vi "COD主界面（列队使用）.vi"() -> (8 "多列列表框":i32(listbox))   [LabVIEW 2016, in "斯坦道CODMn.lvlib"]
uses:
  <vilib>/Analysis/6fits.llb/Curve Fitting Criteria.ctl
  <vilib>/Utility/miscctls.llb/LVPointTypeDef.ctl
  <vilib>/Plasmionique/MB Master/MB_Master_Serial/MB_Master_Serial.lvclass
  D:/Program Files (x86)/National Instruments/LabVIEW 2016/vi.lib/Plasmionique/MB Master/MB_Master/MB_Master.lvclass
  <vilib>/Utility/config.llb/Read Key (Double).vi
  <vilib>/Utility/config.llb/Read Key (U32).vi
  <vilib>/Utility/config.llb/Write Key (Double).vi
  <vilib>/Utility/config.llb/Read Key (I32).vi
  <vilib>/Utility/config.llb/Read Key (Boolean).vi
  <vilib>/Utility/config.llb/Write Key (Boolean).vi
  <vilib>/Utility/config.llb/Write Key (I32).vi
  <vilib>/Waveform/WDTFileIO.llb/Read Waveform from File.vi
  <vilib>/Plasmionique/MB Master/MB Master.lvlib
  <vilib>/ptbypt/NI_PtbyPt.lvlib
  <vilib>/Utility/config.llb/NI_LVConfig.lvlib
  <vilib>/Analysis/NI_AALPro.lvlib
panel:
  out "基本量程(显示)":string
  out "测量模式(显示)":string
  in  "量程切换次数":u8
  in  "CODMn空白测试选择":enum16{"空白测试走纯水管", "空白测试走标样管"}(ring)
  out "数据时间":string
  out "断电排液标记":bool
  in  "测量模式":T1(ring)
  in  "高切低阈值":dbl
  in  "低切高阈值":dbl
  out "COM":string
  in  "启用5":bool
  in  "校准5":bool
  in  "泵滴定数5":dbl
  in  "浓度5":dbl
  in  "启用4":bool
  in  "校准4":bool
  in  "泵滴定数4":dbl
  in  "浓度4":dbl
  out "波形时间":timestamp
  in  "历史波形":bool
  out "滴定数-ORP值":u16[](array[numeric]) caption="数组"
  in  "关闭 3":bool
  in  "滴定曲线":bool
  out "ORP滴定曲线2":u16[](graph)
  in  "跨度液浓度":dbl
  out "空白测试标记":bool
  out "跨度核查标记":bool
  out "启动选择 2":u16(ring) items=["水样测试", "标样核查", "零点核查", "跨度核查", "空白测试", "加标回收", "平行样", "校零", "校标"]
  in  "量程选择":enum16{"低量程", "高量程", "0-2量程"}(ring)
  in  "手动控制":bool
  in  "选用水样":enum16{"葡萄糖", "草酸钠"}(ring)
  in  "方程系数":cluster{"X^2":dbl, "X":dbl, "b":dbl} {"X^2" format="%#.6g"; "b" format="%#.6g"; "X" format="%#.6g"}
  out "多项式系数1":dbl[](array[numeric]) caption="多项式系数"
  out "XY图":cluster{"X Values":dbl[], "Y Values":dbl[]}[](graph)
  in  "模型":enum32{"线性", "多项式"}(ring)
  out "启动时间":timestamp format="%<%Y/%m/%d %H:%M:%S>T"
  in  "自动切换量程":enum16{"关闭", "自动切换测一次", "自动切换测两次"}(ring)
  in  "24H周期设置":bool[](xcontrol)
  in  "关闭 2":bool
  in  "周期设置":bool
  out "文本.文本":string
  out "r^2":dbl format="%.8g"
  out "拟合公式":string
  out "b":dbl format="%#.4g"
  out "K":dbl format="%#.4f"
  out "当前校准":i32
  in  "启用3":bool
  in  "启用2":bool
  in  "启用1":bool
  in  "校准3":bool
  in  "校准2":bool
  in  "校准1":bool
  in  "泵滴定数3":dbl
  in  "泵滴定数2":dbl
  in  "泵滴定数1":dbl
  in  "浓度3":dbl
  in  "浓度2":dbl
  in  "浓度1":dbl
  in  "写入":bool
  out "测量模式数字":i32
  out "零点核查标记":bool
  out "排液故障":bool
  out "进水样超量程":bool
  out "标样核查标记":bool
  out "平行样测量":bool
  out "加标回收测量":bool
  out "质控样测量":bool
  out "待机":bool
  out "校标错误":bool
  out "校零错误":bool
  out "测量错误":bool
  out "草酸钠报警":bool
  out "高锰酸钾报警":bool
  out "加热故障":bool
  out "温控器故障":bool
  out "ORP故障":bool
  out "排液标记":bool
  out "故障标记":bool
  out "校标标记":bool
  out "校零标记":bool
  out "通讯状态":bool
  out "水样测量":bool
  out "读取KB值":bool
  in  "读取":bool
  in  "返回":bool
  in  "校准配置":bool
  in  "修正系数 2":dbl
  in  "浓度 2":dbl
  in  "温度":dbl
  in  "恒温时间":dbl
  in  "基本量程":enum16{"10mg/L", "20mg/L"}(ring)
  in  "水样":dbl
  in  "蒸馏水":dbl
  in  "标液":dbl
  in  "质控样":dbl
  in  "加标回收":dbl
  in  "草酸钠":dbl
  in  "高锰酸钾":dbl
  in  "硫酸":dbl
  in  "零点泵计量数 2":dbl
  in  "标度泵计量数 2":dbl
  out "标度滴定值":dbl
  out "零点滴定值":dbl
  in  "保存":bool
  in  "关闭":bool
  out "测量数据区":T2 {"单位" items=["ug/L", "mg/L", "ppm", "mg/m3", "cm", "ppb", "ug/m3", "%", "nmol/mol", "umol/mol", "MPN/L", "MPN/100ml", "ng/m3", "NTU", "无量纲", "ms/cm", "us/cm", "℃", "mV", "万个/L"]}
  out "仪器时间":timestamp format="%<%Y/%m/%d %H:%M:%S>T"
  out "秒":u16
  out "分":u16
  out "COD浓度（mg/L)":dbl format="%.2g"
  out "进样管":dbl
  out "高锰酸钾":dbl
  out "草酸钠":dbl
  out "硫酸":dbl
  out "ORP显示":dbl
  out "温度":dbl
  out "加热":bool
  out "搅拌":bool
  out "进硫酸":bool
  out "进加标回收样":bool
  out "进质控样":bool
  out "进标液":bool
  out "进蒸馏水":bool
  out "进水样":bool
  out "进草酸钠":bool
  out "进高锰酸钾":bool
  out "定时启动":bool
  in  "启动":bool
  in  "故障清除":bool
  in  "参数配置":bool
  in  "停止":bool
  in  "单步启动":bool
  out "系统时间":timestamp
  in  "时间校准":bool
  in  "枚举":enum16{"读取数据", "写入数据", "读取写入DATABASE", "读取参数"}(ring)
  out "报警簇":T3
  out "Registers":u16[](array[numeric])
  in  "Slave ID":u8=1
  in  "Serial Config":T4={"baud rate (bps)"=115200, "stop bits"=10, "parity"=0, "flow control"=0, "timeout"=1000, "retries"=1} {"stop bits" items=["1.0"=10, "1.5"=15, "2.0"=20]; "flow control" items=["None", "XON/XOFF", "RTS/CTS", "XON/XOFF & RTS/CTS", "DTR/DSR", "XON/XOFF & DTR/DSR"]; "parity" items=["None", "Odd", "Even", "Mark", "Space"]}
  in  "温度 2":dbl
  in  "浓度":dbl
  in  "修正系数":dbl
  in  "标样浓度 2":dbl
  out "模式（受控）":u16
  in  "VISA resource name":refnum<visa-resource-name>="COM4" caption="VISA资源名称"
  # "测量时间："
  # "水样~加标回收"
  # "mV"
  # "℃"
  # "注：遇到加热故障和排液故障时仪器不能正常启动，\n必须排查故障并点击报警清除按钮方可运行。"
  # "mg/L"
  # "校零校标结果"
  # "基本参数设置"
  # "泵计量参数设置"
  # "校零结果："
  # "校零滴定值："
  # "加热恒温温度（℃）："
  # "水样："
  # "高锰酸钾："
  # "校标结果："
  # "标度滴定值："
  # "零点泵计量值："
  # "恒温时间（分钟）："
  # "蒸馏水："
  # "草酸钠："
  # "标度泵计量值："
  # "标准液浓度（mg/L）："
  # "标液："
  # "标样浓度："
  # "硫酸："
  # "修正系数："
  # "质控样："
  # "跨度液浓度："
  # "基本量程（20mg/L可选）："
  # "加标回收样："
  # "是否启用"
  # "泵滴定数"
  # "浓度"
  # "辅\n助\n计\n算\n区"
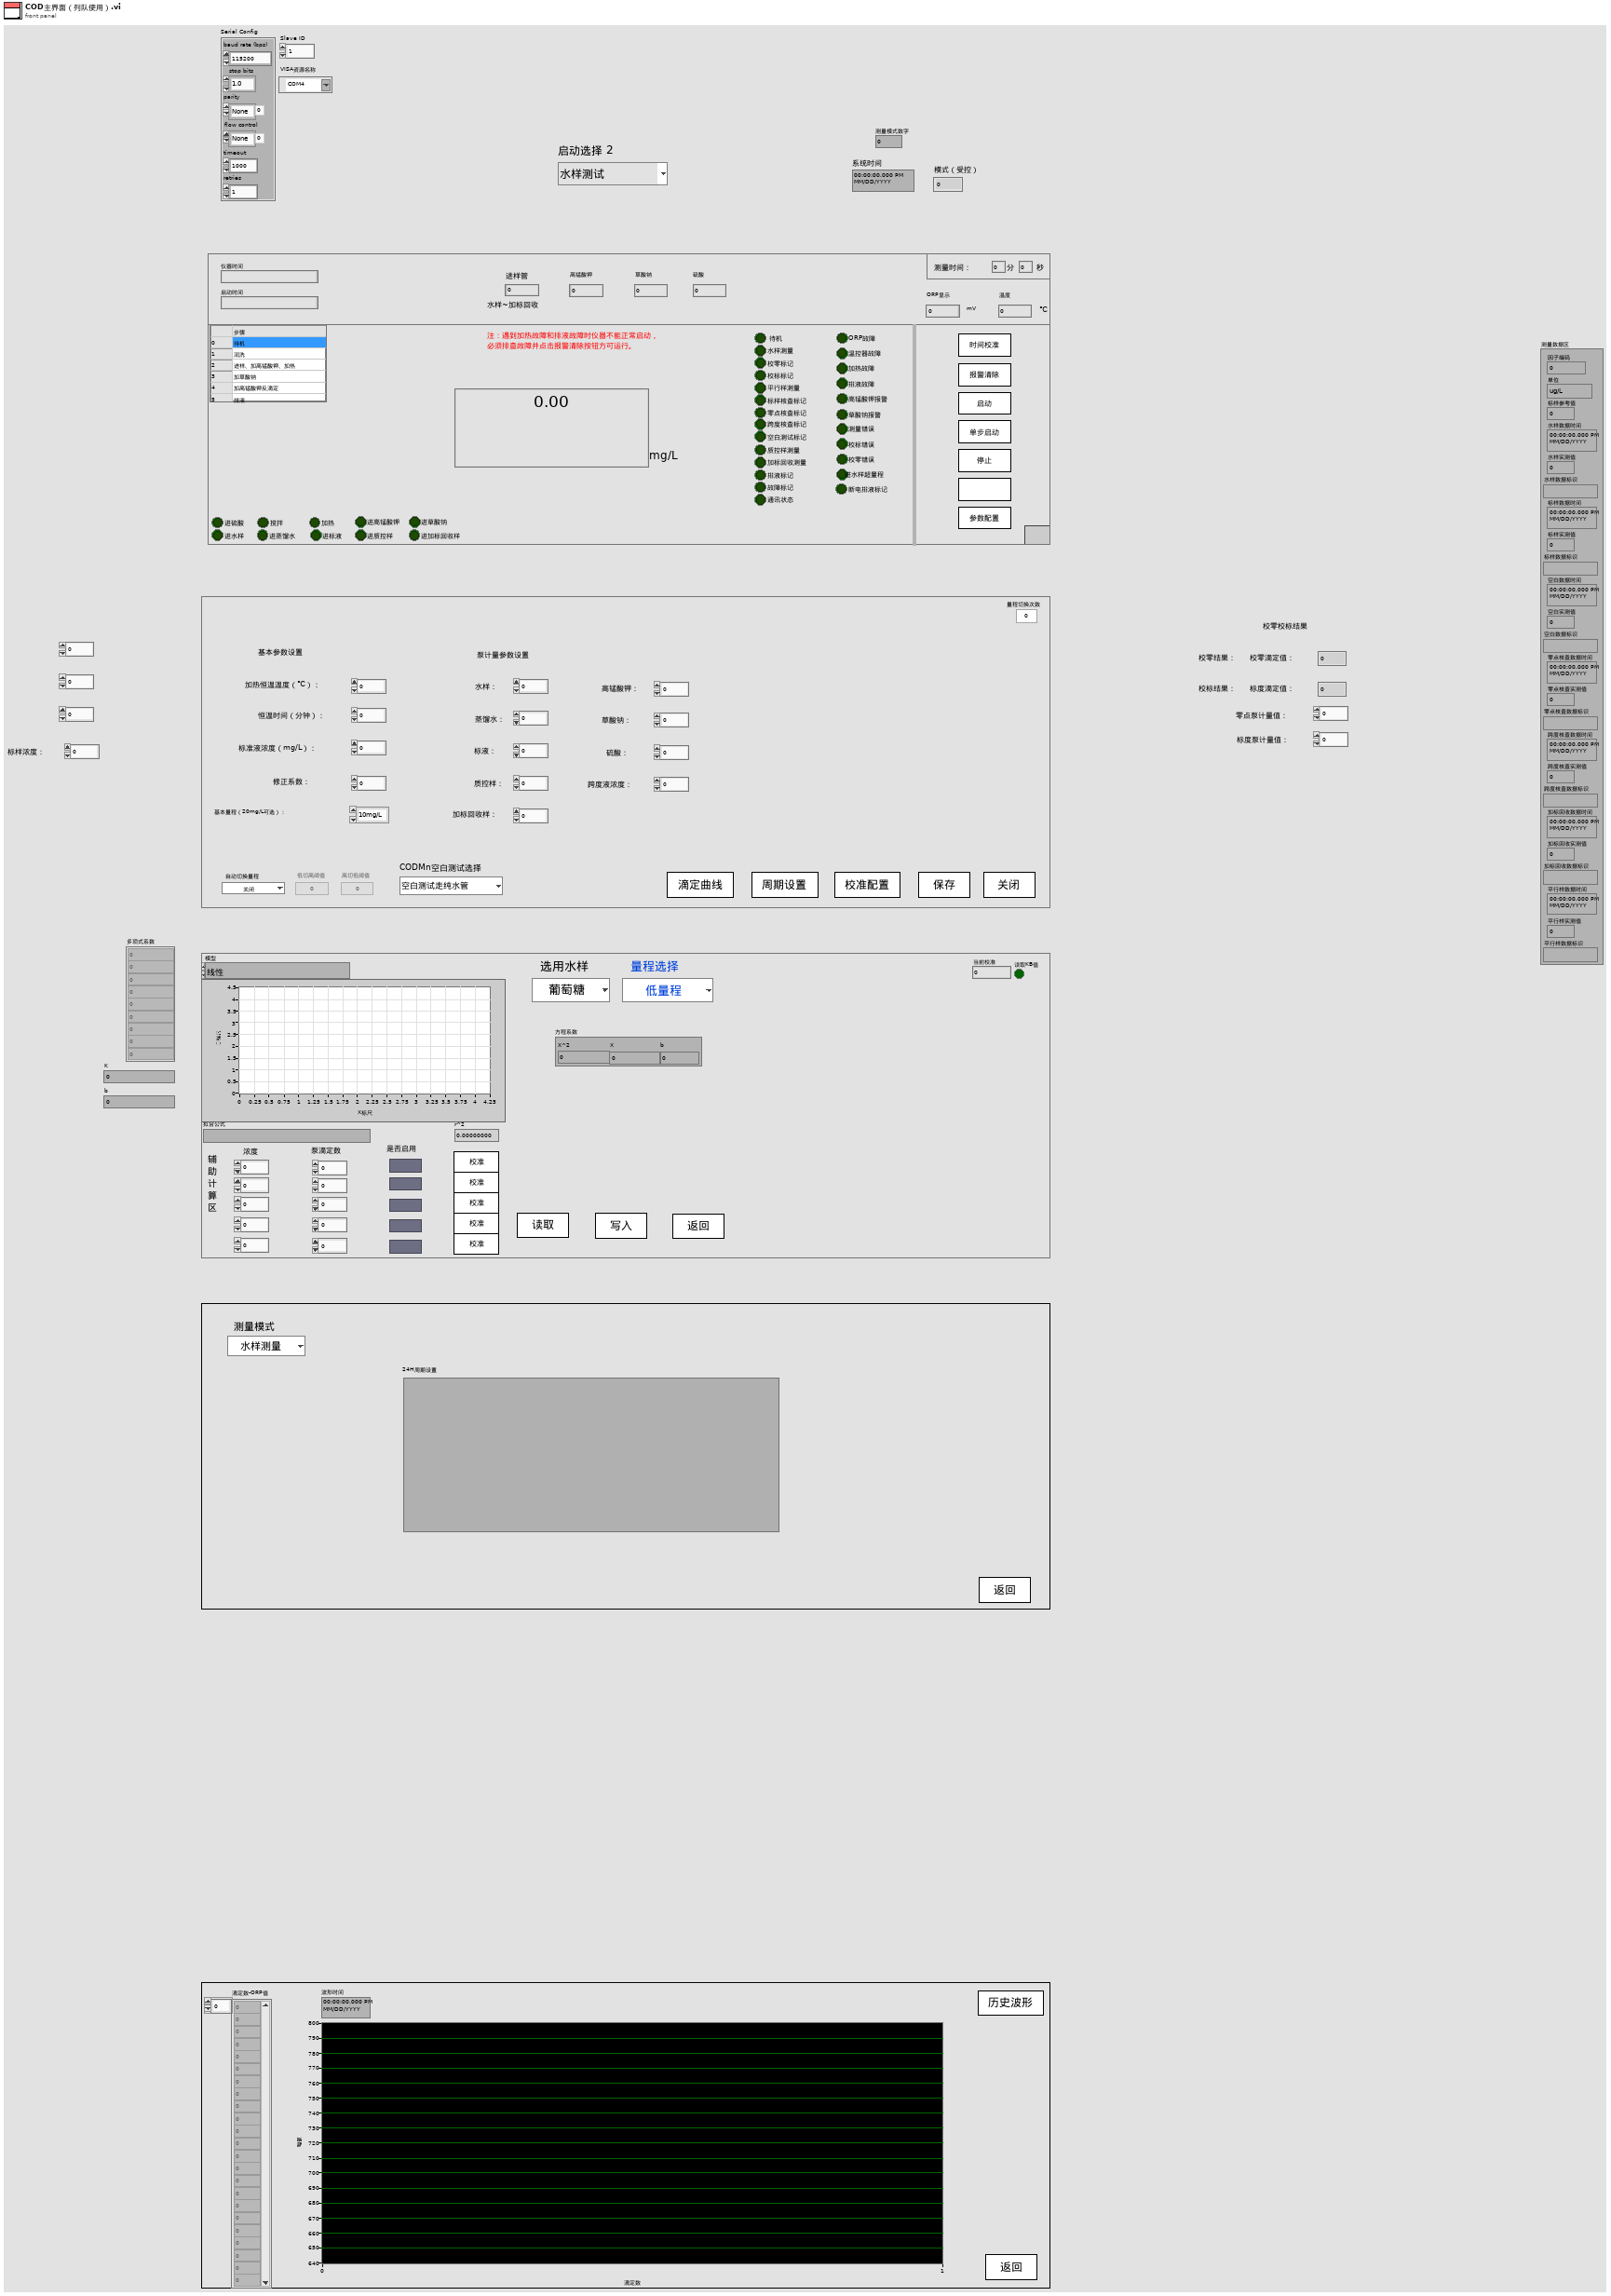
[diagram p1: front panel]
types:
  T1 = enum16{"水样测量", "标样核查", "零点核查", "跨度核查", "空白测试", "加标回收", "平行样", "校零", "校标"}
  T2 = cluster{"因子编码":u32, "单位":u16, "标样参考值":sgl, "水样数据时间":timestamp, "水样实测值":sgl, "水样数据标识":string, "标样数据时间":timestamp, "标样实测值":sgl, "标样数据标识":string, "空白数据时间":timestamp, "空白实测值":sgl, "空白数据标识":string, "零点核查数据时间":timestamp, "零点核查实测值":sgl, "零点核查数据标识":string, "跨度核查数据时间":timestamp, "跨度核查实测值":sgl, "跨度核查数据标识":string, "加标回收数据时间":timestamp, "加标回收实测值":sgl, "加标回收数据标识":string, "平行样数据时间":timestamp, "平行样实测值":sgl, "平行样数据标识":string}
  T3 = cluster{"ORP故障":bool, "温控器故障":bool, "加热故障":bool, "高锰酸钾报警":bool, "草酸钠报警":bool, "测量错误":bool, "校零错误":bool, "校标错误":bool, " 进水样超量程":bool, "排液阀故障":bool}
  T4 = cluster{"baud rate (bps)":u32, "stop bits":u16, "parity":u16, "flow control":u16, "timeout":u32, "retries":i32}
  T5 = cluster{"starting address":u16, "number of holding registers":u16}
  T6 = cluster{"测量模式":enum16{"水样测量", "标样核查", "零点核查", "跨度核查", "空白测试", "加标回收", "平行样", "校零", "校标"}}
  T7 = cluster{"仪器测试类型":enum16{"水样测试", "标样核查", "空白测试", "跨度核查"}, "周期设置类型":enum16{"定点启动", "间隔启动"}, "定时功能启用":bool, "定时间隔":dbl, "24H周期设置":bool[]}
  T8 = typedef "LVDateTimeRec.ctl" = cluster{"秒数的小数部分":dbl, "秒":i32, "分":i32, "时":i32, "日":i32, "月":i32, "年":i32, "天数（周）":i32, "天数（年）":i32, "DST":i32}
  T9 = typedef "LVPointTypeDef.ctl" = cluster{"Horizontal":i16, "Vertical":i16}
  T10 = typedef "NI_LVConfig.lvlib/Config Data RefNum.ctl" = refnum<k1>
  T11 = enum8{"Enabled", "Disabled", "Disabled and Grayed Out"}
  T12 = cluster{"时间标识":timestamp, "参数":string, "日志信息":string, "流程参数":string}
  T13 = cluster{"时间标识":timestamp, "设备":string, "日志信息":string}
  T14 = typedef "NI_AALPro.lvlib/Curve Fitting Criteria.ctl" = u16
  T15 = cluster{"时间标识":timestamp, "设备":string, "日志信息":string, "流程参数":string}
  T16 = cluster{"时间":timestamp, "测量模式":string, "数据类型":string, "检测值":sgl, "单位":string, "数据标识":string, "因子编码":string, "标样参考值":sgl, "ORP-A":sgl, "ORP-B":sgl, "ORP-K":sgl, "COD滴定值":sgl, "高锰酸钾滴定数":sgl, "温度":sgl, "量程":sgl}
  T17 = cluster{"运行模式":enum16{"维护模式", "常规模式", "应急模式", "质控模式"}}
  T18 = cluster{"数组 2[0]":sgl, "数组 2[1]":sgl, "数组 2[2]":sgl, "数组 2[3]":sgl, "数组 2[4]":sgl, "数组 2[5]":sgl, "数组 2[6]":sgl, "数组 2[7]":sgl, "数组 2[8]":sgl}
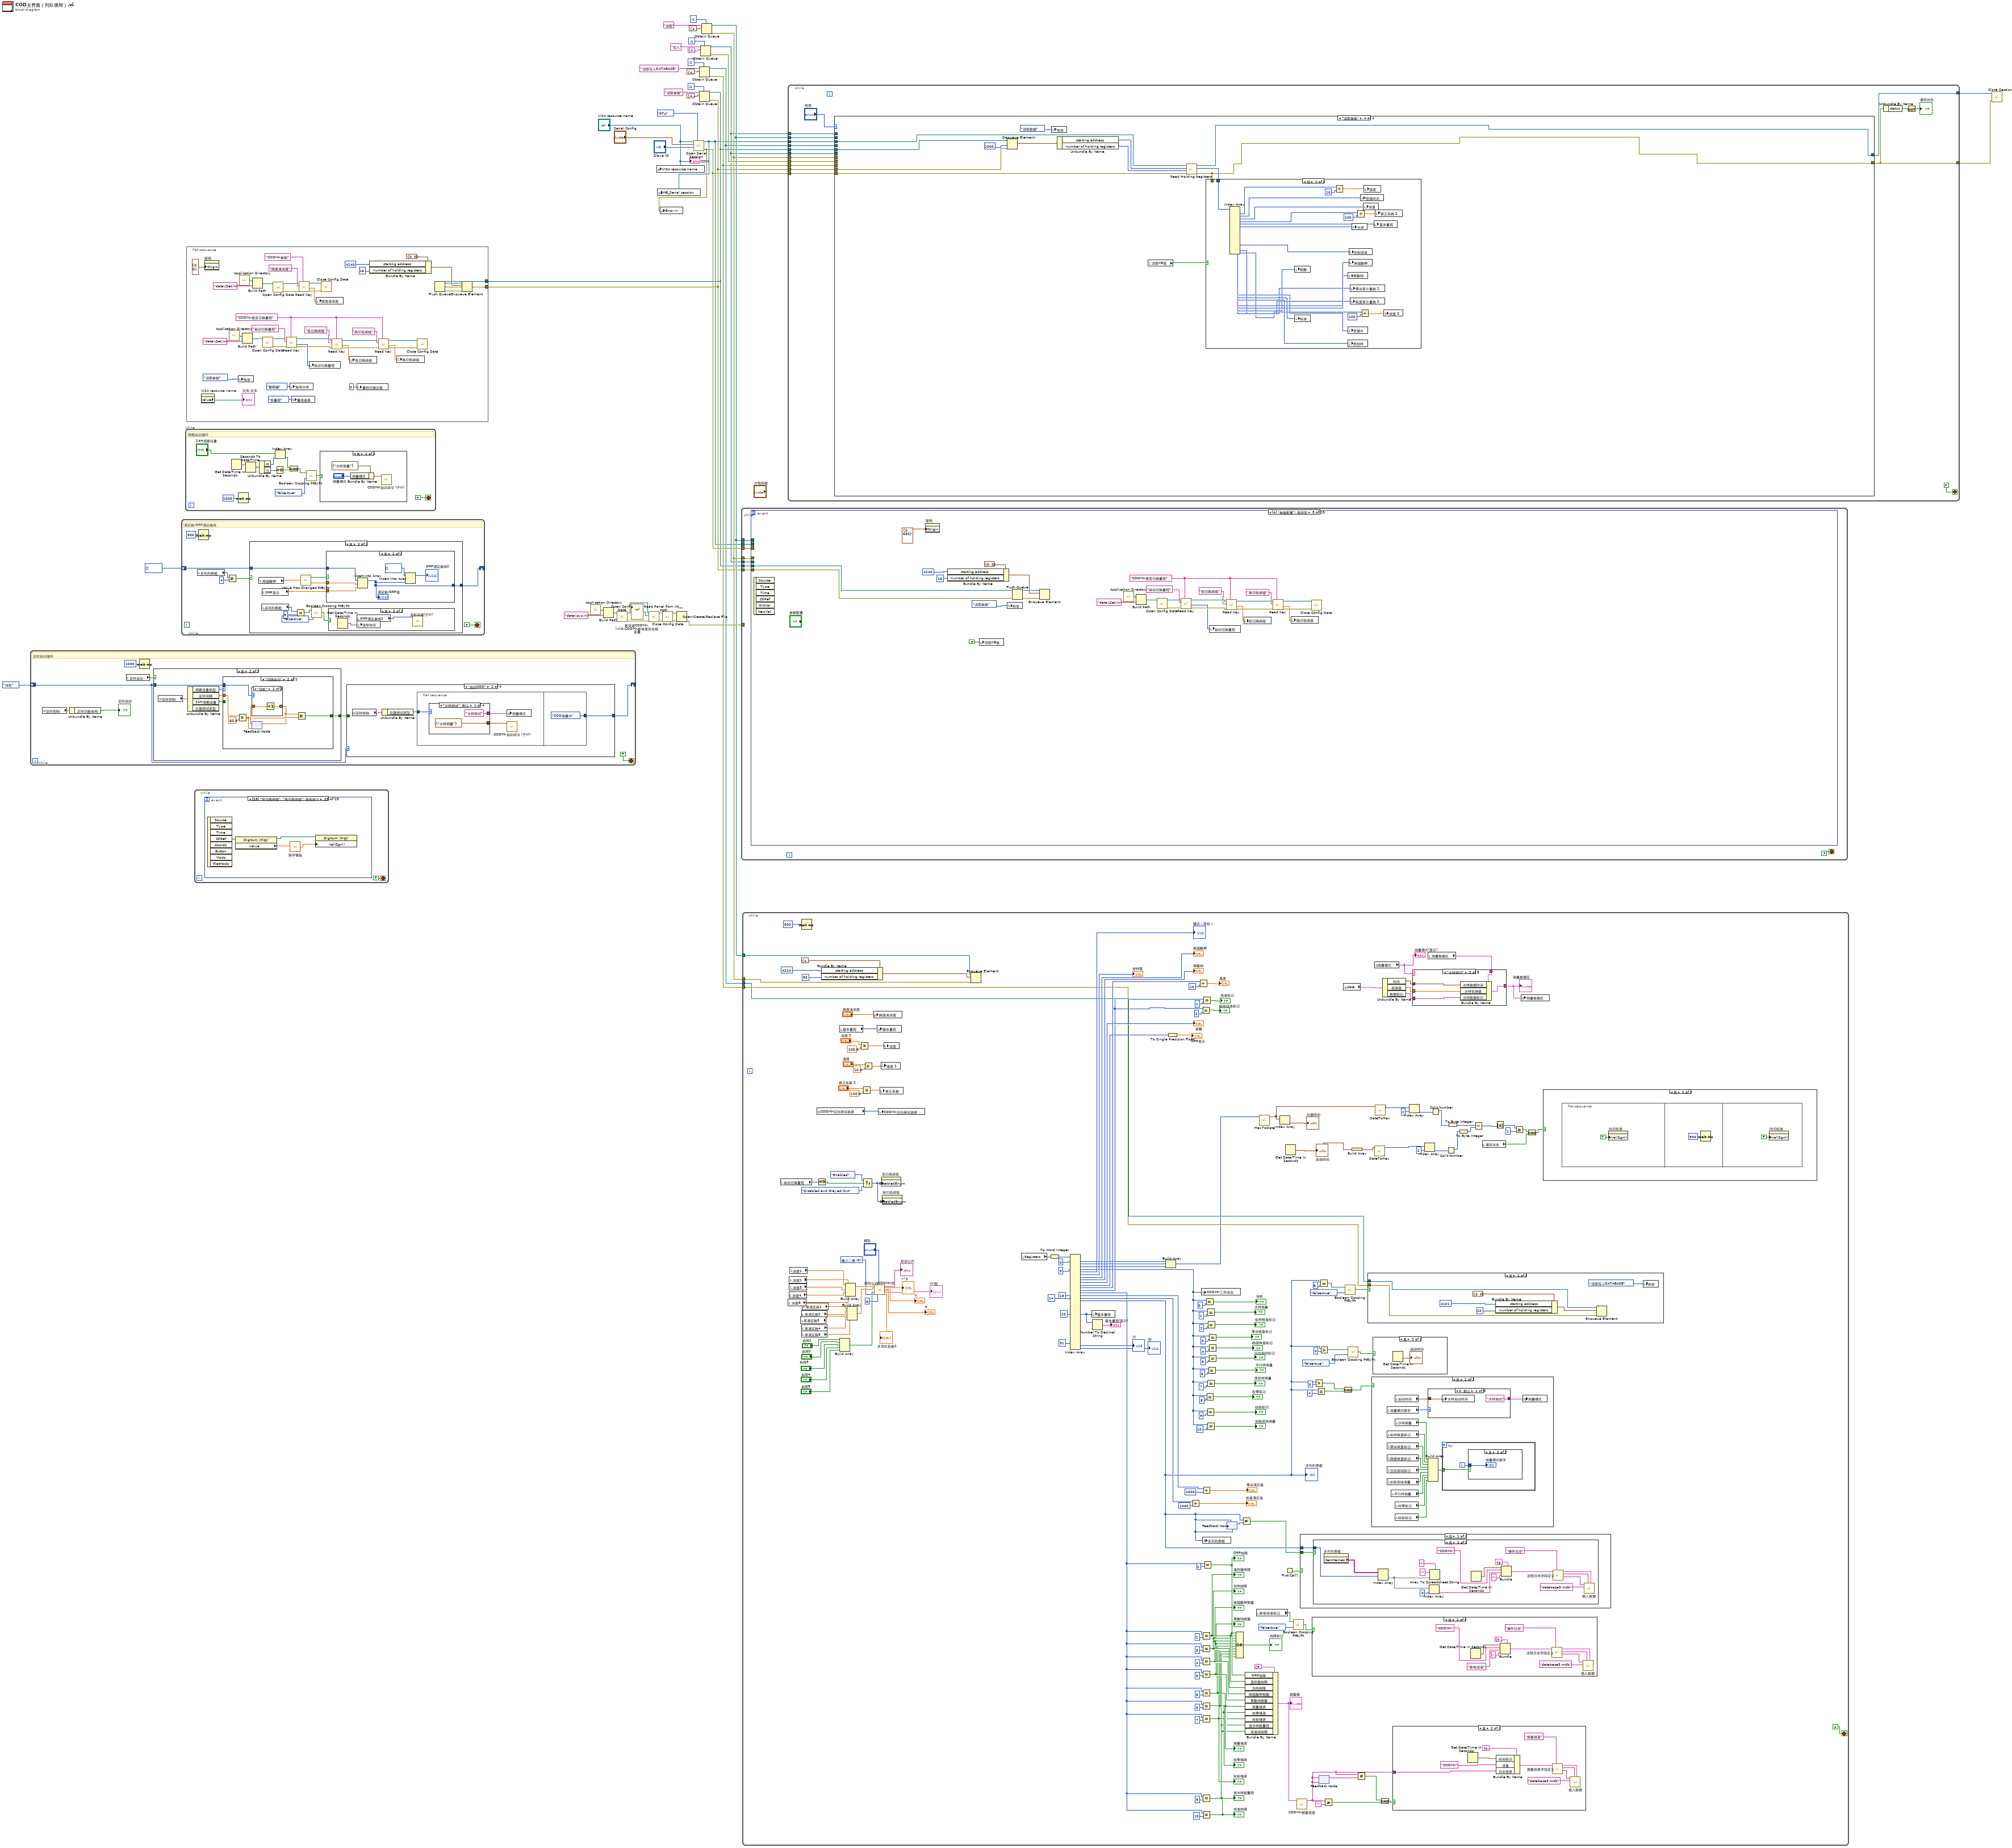
[diagram p0: block diagram]
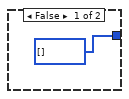
[diagram p2: hidden frame]
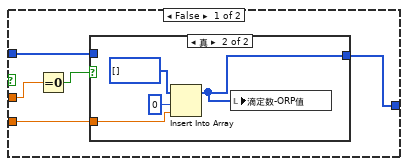
[diagram p4: hidden frame]
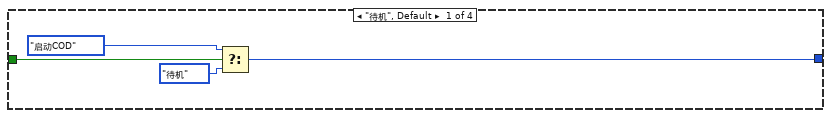
[diagram p7: hidden frame]
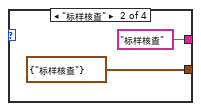
[diagram p8: hidden frame]
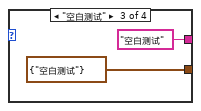
[diagram p9: hidden frame]
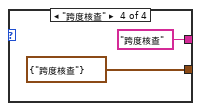
[diagram p10: hidden frame]
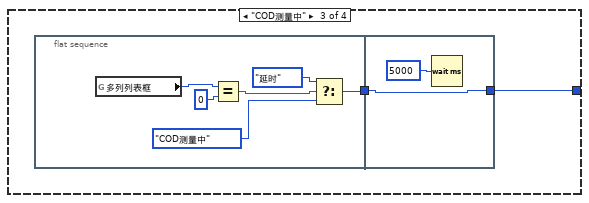
[diagram p11: hidden frame]
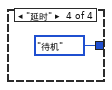
[diagram p12: hidden frame]
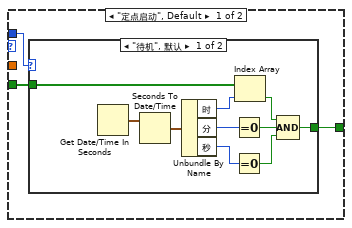
[diagram p14: hidden frame]
diagram:
  n1 = while {
    shift-right: [w47] -> _
    shift-left: enum16{"待机", "启动COD", "COD测量中", "延时"}."待机" -> [w46]
    stop <- FALSE stop-if-true
    # "定时启动循环"
    n2 = global read "CODMn断电保存全局变量.vi" "定时控制"() -> (w43:T7)
    n3 = Unbundle By Name(w43) -> ("定时功能启用"=→"定时启动":bool)
    n4 = local read "定时启动"() -> (w44:bool)
    n5 = Wait (ms)(milliseconds to wait=u32 1000 ("等待时间（毫秒）")) -> ()  [unwired: 1 out]
    n6 = case shown="真" w44 {
      tunnel: w46 -> [_ w82]
      tunnel: [_ w81] -> w45
      frame False {
      }
      frame True {
        n7 = global read "CODMn断电保存全局变量.vi" "定时控制"() -> (w80:T7)
        n8 = Unbundle By Name(w80) -> ("周期设置类型"=w83:enum16{"定点启动", "间隔启动"}, "定时间隔"=w84:dbl, "24H周期设置"=w85:bool[])  [unwired: 1 out]
        n9 = case shown="\"间隔启动\"" w83 {
          tunnel: w84 -> [_ w102]
          tunnel: w85 -> [w88 _]
          tunnel: w82 -> [w86 w105]
          tunnel: [w87 w100] -> w81
          frame "定点启动", Default {
            n10 = case shown="\"待机\", 默认" w86 {
              tunnel: w88 -> [w96 _]
              tunnel: [w89 _] -> w87
              frame "待机", Default {
                n11 = Get Date/Time In Seconds() -> (seconds since 1Jan1904=w98:timestamp)
                n12 = Seconds To Date/Time(time stamp (now)=w98) -> (date time rec=w97:T8)  [unwired: 1 in]
                n13 = Unbundle By Name(w97) -> ("时"=w95:i32, "分"=w93:i32, "秒"=w94:i32)
                n14 = Equal To 0?(x=w93) -> (x = 0?=w91:bool)
                n15 = Equal To 0?(x=w94) -> (x = 0?=w90:bool)
                n16 = Index Array(array=w96, index=w95) -> (element=w92:bool)
                n17 = Compound Arithmetic op=AND ("复合运算")(w92, w91, w90) -> (w89:bool)
              }
              frame "启动COD" {
              }
            }
          }
          frame "间隔启动" {
            n18 = Multiply(x=w102, y=60.0) -> (x*y=w99:dbl)
            n19 = feedback #1(w99) -> (w104:dbl)
            n20 = case shown="\"待机\"" w105 {
              tunnel: w104 -> [_ w107]
              tunnel: [_ w106] -> w103
              frame Default {
              }
              frame "待机" {
                n21 = Increment(x=w107) -> (x+1=w106:dbl)
              }
            }
            n22 = feedback-in #1(w103) -> ()
            n23 = Greater Or Equal?(x=w103, y=w99) -> (x >= y?=w100:bool)
          }
        }
      }
    }
    n24 = case shown="\"启动COD\"" w46 {
      tunnel: [w50 w56 w70 enum16{"待机", "启动COD", "COD测量中", "延时"}."待机"] -> w47
      tunnel: w45 -> [w53 _ _ _]
      frame "待机", Default {
        n25 = Select(t=enum16{"待机", "启动COD", "COD测量中", "延时"}."启动COD", s=w53, f=enum16{"待机", "启动COD", "COD测量中", "延时"}."待机") -> (s? t:f=w50:enum16{"待机", "启动COD", "COD测量中", "延时"})
      }
      frame "启动COD" {
        n26 = global read "CODMn断电保存全局变量.vi" "定时控制"() -> (w54:T7)
        n27 = Unbundle By Name(w54) -> ("仪器测试类型"=w55:enum16{"水样测试", "标样核查", "空白测试", "跨度核查"})
        n28 = flat-sequence {
          tunnel: w55 -> [w59]
          tunnel: [enum16{"待机", "启动COD", "COD测量中", "延时"}."COD测量中"] -> w56
          frame #0 {
            n29 = case shown="\"水样测试\", 默认" w59 {
              tunnel: [T6 {"测量模式"=enum."水样测量"} ("启动测量模式") T6 {"测量模式"=enum."标样核查"} ("启动测量模式") T6 {"测量模式"=enum."空白测试"} ("启动测量模式") T6 {"测量模式"=enum."跨度核查"} ("启动测量模式")] -> w58
              tunnel: ["水样测试" ("测量模式") "标样核查" ("测量模式") "空白测试" ("测量模式") "跨度核查" ("测量模式")] -> w57
              frame "水样测试", Default {
              }
              frame "标样核查" {
              }
              frame "空白测试" {
              }
              frame "跨度核查" {
              }
            }
            n30 = global write "COD测量模式全局.vi" "测量模式"(w57) -> ()
            n31 = call "CODMn启动命令 (子VI).vi"("启动测量模式"=w58) -> ()  [unwired: 11 in]
          }
          frame #1 {
          }
        }
      }
      frame "COD测量中" {
        n32 = flat-sequence {
          tunnel: [w71] -> w69
          tunnel: [w78] -> w70
          tunnel: w69 -> [w78]
          frame #0 {
            n33 = global read "运行时序全局变量.vi" "多列列表框"() -> (w76:i32)
            n34 = Equal?(x=w76, y=0) -> (x = y?=w74:bool)
            n35 = Select(t=enum16{"待机", "启动COD", "COD测量中", "延时"}."延时", s=w74, f=enum16{"待机", "启动COD", "COD测量中", "延时"}."COD测量中") -> (s? t:f=w71:enum16{"待机", "启动COD", "COD测量中", "延时"})
          }
          frame #1 {
            n36 = Wait (ms)(milliseconds to wait=u32 5000 ("等待时间（毫秒）")) -> ()  [unwired: 1 out]
          }
        }
      }
      frame "延时" {
      }
    }
  }
  n37 = while {
    shift-right: [w111] -> _
    shift-left: u16[] [] ("ORP滴定曲线") -> [w112]
    stop <- FALSE stop-if-true
    # "滴定数-ORP滴定曲线"
    n38 = local read "多列列表框"() -> (w110:i32)
    n39 = Wait (ms)(milliseconds to wait=u32 300 ("等待时间（毫秒）")) -> ()  [unwired: 1 out]
    n40 = Greater Or Equal?(x=w110, y=4) -> (x >= y?=w108:bool)
    n41 = case shown="真" w108 {
      tunnel: w112 -> [_ w126]
      tunnel: [u16[] [] ("ORP滴定曲线") w125] -> w111
      frame False {
      }
      frame True {
        n42 = local read "高锰酸钾"() -> (w122:dbl)
        n43 = local read "多列列表框"() -> (w120:i32)
        n44 = local read "ORP显示"() -> (w121:dbl)
        n45 = Equal?(x=w120, y=5) -> (x = y?=w118:bool)
        n46 = call <vilib>:"Value Has Changed PtByPt.vi"("input data point"=w122) -> ("has changed"=w124:bool, "output data point"=w123:dbl)  [unwired: 1 in]
        n47 = call <vilib>:"Boolean Crossing PtByPt.vi"("direction"=enum16{"either", "false-true", "true-false"}."false-true", "input"=w118) -> ("crossing"=w116:bool)  [unwired: 1 in]
        n48 = case shown="真" w124 {
          tunnel: w126 -> [w132 w142]
          tunnel: [w131 w141] -> w125
          tunnel: w123 -> [w133 w140]
          tunnel: w121 -> [w129 w139]
          frame False {
            n49 = Equal To 0?(x=w133) -> (x = 0?=w130:bool)
            n50 = case shown="真" w130 {
              tunnel: [w134 w137] -> w131
              tunnel: w132 -> [w134 _]
              tunnel: w129 -> [_ w136]
              frame False {
              }
              frame True {
                n51 = Insert Into Array(array=u16[] [] ("ORP滴定曲线"), index=0 ("索引"), new element=w136) -> (w137:u16[])
                n52 = local write "滴定数-ORP值"(w137) -> ()
              }
            }
          }
          frame True {
            n53 = Insert Into Array(array=w142, index=w140, new element=w139) -> (w141:u16[])
            "滴定数-ORP值" <- w141
            n54 = Insert Into Array(array=u16[] [] ("ORP滴定曲线"), new element=w141) -> (→"ORP滴定曲线2":u16[])  [unwired: 1 in]
          }
        }
        n55 = case shown="真" w116 {
          frame False {
          }
          frame True {
            n56 = Get Date/Time In Seconds() -> (seconds since 1Jan1904=w127:timestamp)
            n57 = local read "ORP滴定曲线2"() -> (w128:u16[])
            n58 = local write "波形时间"(w127) -> ()
            n59 = call "波形存储(子VI).vi"("ORP滴定曲线"=w128) -> ()  [unwired: 11 in]
          }
        }
      }
    }
  }
  n60 = while "While循环" {
    stop <- FALSE stop-if-true
    # "周期启动循环"
    n61 = Get Date/Time In Seconds() -> (seconds since 1Jan1904=w156:timestamp)
    n62 = Wait (ms)(milliseconds to wait=u32 1000 ("等待时间（毫秒）")) -> ()  [unwired: 1 out]
    n63 = Seconds To Date/Time(time stamp (now)=w156) -> (date time rec=w155:T8)  [unwired: 1 in]
    n64 = Unbundle By Name(w155) -> ("时"=w152:i32, "分"=w154:i32)
    n65 = Equal To 0?(x=w154) -> (x = 0?=w153:bool)
    n66 = Index Array(array="24H周期设置", index=w152) -> (element=w151:bool)
    n67 = And(x=w151, y=w153) -> (x .and. y?=w149:bool)
    n68 = call <vilib>:"Boolean Crossing PtByPt.vi"("direction"=enum16{"either", "false-true", "true-false"}."false-true", "input"=w149) -> ("crossing"=w148:bool)  [unwired: 1 in]
    n69 = case shown="真" w148 {
      frame False {
      }
      frame True {
        n70 = Bundle By Name(cluster=T6 {"测量模式"=enum."水样测量"} ("启动测量模式"), "测量模式"="测量模式") -> (w158:T6)
        n71 = call "CODMn启动命令 (子VI).vi"("启动测量模式"=w158) -> ()  [unwired: 11 in]
      }
    }
  }
  n72 = flat-sequence {
    tunnel: w15 -> [w183]
    tunnel: w14 -> [w182]
    frame #0 {
      w175 = "CODMn是否切换量程" ("key")
      n73 = property on="VISA resource name" class="VISAName"() -> ("Value"=→"文本.文本":refnum<visa-resource-name>)  [unwired: 2 in, 2 out]
      n74 = property on="窗格" class="Pane"("Origin"=T9 {"Horizontal"=0, "Vertical"=0} ("原点")) -> ()  [unwired: 2 in, 2 out]
      n75 = call <vilib>:"Application Directory.vi"() -> ("Application Directory"=w167:path)
      n76 = local write "枚举"(enum16{"读取数据", "写入数据", "读取写入DATABASE", "读取参数"}."读取参数" ("枚举")) -> ()
      n77 = call <vilib>:"Application Directory.vi"() -> ("Application Directory"=w191:path)
      n78 = Build Path(base path=w167, name or relative path="data\\Set.ini" ("名称或相对路径")) -> (appended path=w169:path)
      n79 = Build Path(base path=w191, name or relative path="data\\Set.ini" ("名称或相对路径")) -> (appended path=w193:path)
      n80 = call <vilib>:"Open Config Data.vi"("configuration file path"=w169) -> ("error out"=w166:errorcluster, "refnum"=w165:T10)  [unwired: 8 in, 1 out]
      n81 = call <vilib>:"Open Config Data.vi"("configuration file path"=w193) -> ("error out"=w197:errorcluster, "refnum"=w196:T10)  [unwired: 8 in, 1 out]
      n82 = call-poly <vilib>:"Read Key.vi"("section"=w175, "error in (no error)"=w166, "key"="自动切换量程", "refnum"=w165) -> ("error out"=w172:errorcluster, "value"=w161:u32, "refnum out"=w171:T10)  [unwired: 4 in, 1 out]
      n83 = local write "选用水样"(enum16{"葡萄糖", "草酸钠"}."葡萄糖" ("选用水样")) -> ()
      n84 = local write "量程选择"(enum16{"低量程", "高量程", "0-2量程"}."低量程" ("量程选择")) -> ()
      n85 = call-poly <vilib>:"Read Key.vi"("section"="CODMn参数" ("key"), "error in (no error)"=w197, "key"="跨度液浓度", "refnum"=w196) -> ("error out"=w199:errorcluster, "value"=w200:dbl, "refnum out"=w198:T10)  [unwired: 4 in, 1 out]
      n86 = local write "自动切换量程"(w161) -> ()
      n87 = local write "跨度液浓度"(w200) -> ()
      n88 = call <vilib>:"Close Config Data.vi"("error in (no error)"=w199, "refnum"=w198) -> ()  [unwired: 8 in, 2 out]
      n89 = call-poly <vilib>:"Read Key.vi"("section"=w175, "error in (no error)"=w172, "key"="低切高阈值", "refnum"=w171) -> ("error out"=w174:errorcluster, "value"=w180:dbl, "refnum out"=w173:T10)  [unwired: 4 in, 1 out]
      n90 = local write "低切高阈值"(w180) -> ()
      n91 = local write "量程切换次数"(u8 0 ("量程切换次数")) -> ()
      n92 = Bundle By Name(cluster=T5 {"starting address"=0, "number of holding registers"=0}, "starting address"=u16 4240, "number of holding registers"=u16 16) -> (w190:T5)
      n93 = call-poly <vilib>:"Read Key.vi"("section"=w175, "error in (no error)"=w174, "key"="高切低阈值", "refnum"=w173) -> ("error out"=w177:errorcluster, "value"=w181:dbl, "refnum out"=w176:T10)  [unwired: 4 in, 1 out]
      n94 = local write "高切低阈值"(w181) -> ()
      n95 = call <vilib>:"Close Config Data.vi"("error in (no error)"=w177, "refnum"=w176) -> ()  [unwired: 8 in, 2 out]
      n96 = Flush Queue(queue=w183, error in (no error)=w182) -> (queue out=w186:refnum<queue>, error out=w185:errorcluster)  [unwired: 1 out]
      n97 = Enqueue Element(queue=w186, element=w190, error in (no error)=w185) -> ()  [unwired: 1 in, 3 out]
    }
  }
  n98 = while {
    stop <- FALSE stop-if-true
    n99 = event shown="[28] \"低切高阈值\", \"高切低阈值\": 鼠标按下" {
      selector: _ -> [_ _ _ _ _ _ _ _ _ _ _ _ _ _ _ _ _ _ _ _ _ _ _ _ _ _ _ _ _]
      dyn-events: _ -> [_ _ _ _ _ _ _ _ _ _ _ _ _ _ _ _ _ _ _ _ _ _ _ _ _ _ _ _ _]
      timeout: _ -> [_ _ _ _ _ _ _ _ _ _ _ _ _ _ _ _ _ _ _ _ _ _ _ _ _ _ _ _ _]
      event Timeout {
        n100 = event-data() -> ()  [unwired: 1 in, 3 out]
      }
      event "温度": Mouse Down {
        n101 = event-data() -> ()  [unwired: 1 in, 8 out]
        n102 = local read "温度"() -> (w204:dbl)
        n103 = call "数字键盘.vi"("OldNumber"=w204) -> ("NewNumber"=w203:sgl)
        n104 = local write "温度"(w203) -> ()
      }
      event "恒温时间": Mouse Down {
        n105 = event-data() -> ()  [unwired: 1 in, 8 out]
        n106 = local read "恒温时间"() -> (w205:dbl)
        n107 = call "数字键盘.vi"("OldNumber"=w205) -> ("NewNumber"=w206:sgl)
        n108 = local write "恒温时间"(w206) -> ()
      }
      event "浓度 2": Mouse Down {
        n109 = event-data() -> ()  [unwired: 1 in, 8 out]
        n110 = local read "浓度 2"() -> (w208:dbl)
        n111 = call "数字键盘.vi"("OldNumber"=w208) -> ("NewNumber"=w207:sgl)
        n112 = local write "浓度 2"(w207) -> ()
      }
      event "修正系数 2": Mouse Down {
        n113 = event-data() -> ()  [unwired: 1 in, 8 out]
        n114 = local read "修正系数 2"() -> (w209:dbl)
        n115 = call "数字键盘.vi"("OldNumber"=w209) -> ("NewNumber"=w210:sgl)
        n116 = local write "修正系数 2"(w210) -> ()
      }
      event "水样": Mouse Down {
        n117 = event-data() -> ()  [unwired: 1 in, 8 out]
        n118 = local read "水样"() -> (w211:dbl)
        n119 = call "数字键盘.vi"("OldNumber"=w211) -> ("NewNumber"=w212:sgl)
        n120 = local write "水样"(w212) -> ()
      }
      event "蒸馏水": Mouse Down {
        n121 = event-data() -> ()  [unwired: 1 in, 8 out]
        n122 = local read "蒸馏水"() -> (w213:dbl)
        n123 = call "数字键盘.vi"("OldNumber"=w213) -> ("NewNumber"=w214:sgl)
        n124 = local write "蒸馏水"(w214) -> ()
      }
      event "标液": Mouse Down {
        n125 = event-data() -> ()  [unwired: 1 in, 8 out]
        n126 = local read "标液"() -> (w215:dbl)
        n127 = call "数字键盘.vi"("OldNumber"=w215) -> ("NewNumber"=w216:sgl)
        n128 = local write "标液"(w216) -> ()
      }
      event "质控样": Mouse Down {
        n129 = event-data() -> ()  [unwired: 1 in, 8 out]
        n130 = local read "质控样"() -> (w217:dbl)
        n131 = call "数字键盘.vi"("OldNumber"=w217) -> ("NewNumber"=w218:sgl)
        n132 = local write "质控样"(w218) -> ()
      }
      event "加标回收": Mouse Down {
        n133 = event-data() -> ()  [unwired: 1 in, 8 out]
        n134 = local read "加标回收"() -> (w219:dbl)
        n135 = call "数字键盘.vi"("OldNumber"=w219) -> ("NewNumber"=w220:sgl)
        n136 = local write "加标回收"(w220) -> ()
      }
      event "草酸钠": Mouse Down {
        n137 = event-data() -> ()  [unwired: 1 in, 8 out]
        n138 = local read "草酸钠"() -> (w221:dbl)
        n139 = call "数字键盘.vi"("OldNumber"=w221) -> ("NewNumber"=w222:sgl)
        n140 = local write "草酸钠"(w222) -> ()
      }
      event "高锰酸钾": Mouse Down {
        n141 = event-data() -> ()  [unwired: 1 in, 8 out]
        n142 = local read "高锰酸钾"() -> (w223:dbl)
        n143 = call "数字键盘.vi"("OldNumber"=w223) -> ("NewNumber"=w224:sgl)
        n144 = local write "高锰酸钾"(w224) -> ()
      }
      event "硫酸": Mouse Down {
        n145 = event-data() -> ()  [unwired: 1 in, 8 out]
        n146 = local read "硫酸"() -> (w225:dbl)
        n147 = call "数字键盘.vi"("OldNumber"=w225) -> ("NewNumber"=w226:sgl)
        n148 = local write "硫酸"(w226) -> ()
      }
      event "零点泵计量数 2": Mouse Down {
        n149 = event-data() -> ()  [unwired: 1 in, 8 out]
        n150 = local read "零点泵计量数 2"() -> (w227:dbl)
        n151 = call "数字键盘.vi"("OldNumber"=w227) -> ("NewNumber"=w228:sgl)
        n152 = local write "零点泵计量数 2"(w228) -> ()
      }
      event "标度泵计量数 2": Mouse Down {
        n153 = event-data() -> ()  [unwired: 1 in, 8 out]
        n154 = local read "标度泵计量数 2"() -> (w229:dbl)
        n155 = call "数字键盘.vi"("OldNumber"=w229) -> ("NewNumber"=w230:sgl)
        n156 = local write "标度泵计量数 2"(w230) -> ()
      }
      event "标样浓度 2": Mouse Down {
        n157 = event-data() -> ()  [unwired: 1 in, 8 out]
        n158 = local read "标样浓度 2"() -> (w231:dbl)
        n159 = call "数字键盘.vi"("OldNumber"=w231) -> ("NewNumber"=w232:sgl)
        n160 = local write "标样浓度 2"(w232) -> ()
      }
      event "浓度1": Mouse Down {
        n161 = event-data() -> ()  [unwired: 1 in, 8 out]
        n162 = local read "浓度1"() -> (w234:dbl)
        n163 = call "数字键盘.vi"("OldNumber"=w234) -> ("NewNumber"=w233:sgl)
        n164 = property on="浓度1" class="DigNum (严格)"("Val(Sgnl)"=w233) -> ()  [unwired: 2 in, 2 out]
      }
      event "浓度2": Mouse Down {
        n165 = event-data() -> ()  [unwired: 1 in, 8 out]
        n166 = local read "浓度2"() -> (w236:dbl)
        n167 = call "数字键盘.vi"("OldNumber"=w236) -> ("NewNumber"=w235:sgl)
        n168 = property on="浓度2" class="DigNum (严格)"("Val(Sgnl)"=w235) -> ()  [unwired: 2 in, 2 out]
      }
      event "浓度3": Mouse Down {
        n169 = event-data() -> ()  [unwired: 1 in, 8 out]
        n170 = local read "浓度3"() -> (w238:dbl)
        n171 = call "数字键盘.vi"("OldNumber"=w238) -> ("NewNumber"=w237:sgl)
        n172 = property on="浓度3" class="DigNum (严格)"("Val(Sgnl)"=w237) -> ()  [unwired: 2 in, 2 out]
      }
      event "浓度4": Mouse Down {
        n173 = event-data() -> ()  [unwired: 1 in, 8 out]
        n174 = local read "浓度4"() -> (w240:dbl)
        n175 = call "数字键盘.vi"("OldNumber"=w240) -> ("NewNumber"=w239:sgl)
        n176 = property on="浓度4" class="DigNum (严格)"("Val(Sgnl)"=w239) -> ()  [unwired: 2 in, 2 out]
      }
      event "浓度5": Mouse Down {
        n177 = event-data() -> ()  [unwired: 1 in, 8 out]
        n178 = local read "浓度5"() -> (w242:dbl)
        n179 = call "数字键盘.vi"("OldNumber"=w242) -> ("NewNumber"=w241:sgl)
        n180 = property on="浓度5" class="DigNum (严格)"("Val(Sgnl)"=w241) -> ()  [unwired: 2 in, 2 out]
      }
      event "跨度液浓度": Mouse Down {
        n181 = event-data() -> ()  [unwired: 1 in, 8 out]
        n182 = local read "跨度液浓度"() -> (w244:dbl)
        n183 = call "数字键盘.vi"("OldNumber"=w244) -> ("NewNumber"=w243:sgl)
        n184 = property on="跨度液浓度" class="DigNum (严格)"("Val(Sgnl)"=w243) -> ()  [unwired: 2 in, 2 out]
      }
      event "跨度液浓度": Value Change {
        n185 = event-data() -> ()  [unwired: 1 in, 6 out]
        n186 = call <vilib>:"Application Directory.vi"() -> ("Application Directory"=w248:path)
        n187 = Build Path(base path=w248, name or relative path="data\\Set.ini" ("名称或相对路径")) -> (appended path=w250:path)
        n188 = local read "跨度液浓度"() -> (w245:dbl)
        n189 = call <vilib>:"Open Config Data.vi"("configuration file path"=w250) -> ("error out"=w252:errorcluster, "refnum"=w251:T10)  [unwired: 8 in, 1 out]
        n190 = call-poly <vilib>:"Write Key.vi"("section"="CODMn参数" ("key"), "error in (no error)"=w252, "value"=w245, "key"="跨度液浓度", "refnum"=w251) -> ("error out"=w254:errorcluster, "refnum out"=w253:T10)  [unwired: 4 in, 1 out]
        n191 = call <vilib>:"Close Config Data.vi"("error in (no error)"=w254, "refnum"=w253) -> ()  [unwired: 8 in, 2 out]
      }
      event "泵滴定数1": Mouse Down {
        n192 = event-data() -> ()  [unwired: 1 in, 8 out]
        n193 = local read "泵滴定数1"() -> (w256:dbl)
        n194 = call "数字键盘.vi"("OldNumber"=w256) -> ("NewNumber"=w255:sgl)
        n195 = property on="泵滴定数1" class="DigNum (严格)"("Val(Sgnl)"=w255) -> ()  [unwired: 2 in, 2 out]
      }
      event "泵滴定数2": Mouse Down {
        n196 = event-data() -> ()  [unwired: 1 in, 8 out]
        n197 = local read "泵滴定数2"() -> (w258:dbl)
        n198 = call "数字键盘.vi"("OldNumber"=w258) -> ("NewNumber"=w257:sgl)
        n199 = property on="泵滴定数2" class="DigNum (严格)"("Val(Sgnl)"=w257) -> ()  [unwired: 2 in, 2 out]
      }
      event "泵滴定数3": Mouse Down {
        n200 = event-data() -> ()  [unwired: 1 in, 8 out]
        n201 = local read "泵滴定数3"() -> (w260:dbl)
        n202 = call "数字键盘.vi"("OldNumber"=w260) -> ("NewNumber"=w259:sgl)
        n203 = property on="泵滴定数3" class="DigNum (严格)"("Val(Sgnl)"=w259) -> ()  [unwired: 2 in, 2 out]
      }
      event "泵滴定数4": Mouse Down {
        n204 = event-data() -> ()  [unwired: 1 in, 8 out]
        n205 = local read "泵滴定数4"() -> (w262:dbl)
        n206 = call "数字键盘.vi"("OldNumber"=w262) -> ("NewNumber"=w261:sgl)
        n207 = property on="泵滴定数4" class="DigNum (严格)"("Val(Sgnl)"=w261) -> ()  [unwired: 2 in, 2 out]
      }
      event "泵滴定数5": Mouse Down {
        n208 = event-data() -> ()  [unwired: 1 in, 8 out]
        n209 = local read "泵滴定数5"() -> (w264:dbl)
        n210 = call "数字键盘.vi"("OldNumber"=w264) -> ("NewNumber"=w263:sgl)
        n211 = property on="泵滴定数5" class="DigNum (严格)"("Val(Sgnl)"=w263) -> ()  [unwired: 2 in, 2 out]
      }
      event "低切高阈值", "高切低阈值": Mouse Down {
        n212 = event-data() -> ("CtlRef"=w268:refnum<vi>)  [unwired: 1 in, 7 out]
        n213 = property class="DigNum (严格)"(reference=w268) -> (reference out=w267:refnum<vi>, "Value"=w266:dbl)  [unwired: 1 in, 1 out]
        n214 = call "数字键盘.vi"("OldNumber"=w266) -> ("NewNumber"=w265:sgl)
        n215 = property class="DigNum (严格)"(reference=w267, "Val(Sgnl)"=w265) -> ()  [unwired: 1 in, 2 out]
      }
    }
  }
  n216 = call <vilib>:"Application Directory.vi"() -> ("Application Directory"=w4:path)
  n217 = Build Path(base path=w4, name or relative path="data\\sys.ini" ("名称或相对路径")) -> (appended path=w6:path)
  n218 = call <vilib>:"Open Config Data.vi"("configuration file path"=w6) -> ("error out"=w10:errorcluster, "refnum"=w7:T10)  [unwired: 8 in, 1 out]
  n219 = vi-ref "斯坦道CODMn.lvlib:CODMn断电保存全局变量.vi"() -> (w8:refnum<vi>)
  n220 = call <userlib>:"Read Panel from INI__ogtk.vi"("error in (no error)"=w10, "VI ref"=w8, "refnum"=w7) -> ("error out"=w11:errorcluster, "refnum out"=w9:T10)  [unwired: 7 in]
  n221 = global write "COD浓度全局变量.vi" "VISA resource name"("VISA resource name") -> ()
  n222 = call <vilib>:"Close Config Data.vi"("error in (no error)"=w11, "refnum"=w9) -> ("error out"=w12:errorcluster, "file path"=w13:path)  [unwired: 8 in]
  n223 = Open/Create/Replace File(file path (use dialog)=w13, error in=w12) -> (error out=w3:errorcluster)  [unwired: 4 in, 2 out]
  n224 = call <vilib>:"Open Serial Session.vi"("Mode (RTU)"=enum16{"RTU", "ASCII"}."RTU", "Slave ID"="Slave ID", "Serial Config"="Serial Config", "VISA Resource"="VISA resource name") -> ("Error out"=w1:errorcluster, "MB_Serial session"=w2:refnum<class "MB_Master_Serial.lvclass">)  [unwired: 6 in]
  n225 = global write "COD浓度全局变量.vi" "MB_Serial session"(w2) -> ()
  n226 = global write "COD浓度全局变量.vi" "Error in"(w1) -> ()
  n227 = Obtain Queue(max queue size (-1, unlimited)=-1 ("队列最大值（-1，无限）"), name (unnamed)="读取写入DATABASE" ("名称（未命名）"), element data type=T5 {"starting address"=4224, "number of holding registers"=16}) -> (queue out=w22:refnum<queue>, error out=w21:errorcluster)  [unwired: 2 in, 1 out]
  n228 = Obtain Queue(max queue size (-1, unlimited)=-1 ("队列最大值（-1，无限）"), name (unnamed)="读取参数" ("名称（未命名）"), element data type=T5 {"starting address"=4224, "number of holding registers"=16}) -> (queue out=w15:refnum<queue>, error out=w14:errorcluster)  [unwired: 2 in, 1 out]
  n229 = Obtain Queue(max queue size (-1, unlimited)=-1 ("队列最大值（-1，无限）"), name (unnamed)="写入" ("名称（未命名）"), element data type=cluster{"starting address":u16, "values":u16[]} {"starting address"=4272, "values"=[]}) -> (queue out=w18:refnum<queue>, error out=w20:errorcluster)  [unwired: 2 in, 1 out]
  n230 = Obtain Queue(max queue size (-1, unlimited)=-1 ("队列最大值（-1，无限）"), name (unnamed)="读取" ("名称（未命名）"), element data type=T5 {"starting address"=4224, "number of holding registers"=16}) -> (queue out=w32:refnum<queue>, error out=w31:errorcluster)  [unwired: 2 in, 1 out]
  n231 = while {
    tunnel: w32 -> [w276]
    tunnel: w31 -> [w275]
    tunnel: w18 -> [w274]
    tunnel: w15 -> [w273]
    tunnel: w14 -> [w272]
    tunnel: w2 -> [w270]
    tunnel: w1 -> [w269]
    tunnel: w3 -> [_]
    stop <- FALSE stop-if-true
    n232 = event shown="[4] \"参数配置\": 值改变" {
      selector: _ -> [_ _ _ _ _ _ _ _ _ _ _ _ _ _ _ _ _ _ _ _ _ _ _ _ _]
      dyn-events: _ -> [_ _ _ _ _ _ _ _ _ _ _ _ _ _ _ _ _ _ _ _ _ _ _ _ _]
      timeout: _ -> [_ _ _ _ _ _ _ _ _ _ _ _ _ _ _ _ _ _ _ _ _ _ _ _ _]
      tunnel: w276 -> [_ _ _ _ _ _ _ _ _ _ _ _ _ _ _ _ _ _ _ _ _ _ _ _ _]
      tunnel: w275 -> [_ _ _ _ _ _ _ _ _ _ _ _ _ _ _ _ _ _ _ _ _ _ _ _ _]
      tunnel: w274 -> [w284 w317 w354 _ _ w396 _ _ _ _ _ _ _ w756 w770 _ _ w807 _ _ _ _ w994 _ _]
      tunnel: w273 -> [_ _ _ _ w387 _ _ _ _ _ _ _ _ _ _ _ _ _ _ _ _ w986 _ _ _]
      tunnel: w272 -> [_ _ _ _ w386 _ _ _ _ _ _ _ _ _ _ _ _ _ _ _ _ w985 _ _ _]
      tunnel: w270 -> [_ _ _ w360 _ _ _ _ _ _ _ _ w755 _ _ _ _ _ _ _ _ _ _ _ _]
      tunnel: w269 -> [_ _ _ w359 _ _ _ _ _ _ _ _ w754 _ _ _ _ _ _ _ _ _ _ _ _]
      event "单步启动": Mouse Down {
        n233 = event-data() -> ()  [unwired: 1 in, 8 out]
        n234 = call "单步启动选择对话框.vi"() -> ("启动选择2"=w277:u16)  [unwired: 10 in, 1 out]
        n235 = case shown="3" w277 {
          tunnel: [u16 4610 ("address") u16 4610 ("address") u16 4610 ("address") u16 4610 ("address") u16 4610 ("address") u16 4610 ("address") u16 4610 ("address") u16 4610 ("address") u16 4610 ("address") u16 4610 ("address") u16 4610 ("address") u16 4610 ("address") u16 4610 ("address")] -> w283
          tunnel: [u16 1 ("address") u16 2 ("address") u16 3 ("address") u16 4 ("address") u16 5 ("address") u16 6 ("address") u16 7 ("address") u16 8 ("address") u16 9 ("holding register value") u16 10 ("holding register value") u16 11 ("holding register value") u16 12 ("address") u16 0 ("address")] -> w280
          frame 0 {
          }
          frame 1 {
          }
          frame 2 {
          }
          frame 3 {
          }
          frame 4 {
          }
          frame 5 {
          }
          frame 6 {
          }
          frame 7 {
          }
          frame 8 {
          }
          frame 9 {
          }
          frame 10 {
          }
          frame 11 {
          }
          frame 12, Default {
          }
        }
        n236 = local write "枚举"(enum16{"读取数据", "写入数据", "读取写入DATABASE", "读取参数"}."写入数据" ("枚举")) -> ()
        n237 = Insert Into Array(array=u16[] [] ("values"), index=0 ("索引"), new element=w280) -> (w279:u16[])
        n238 = Bundle By Name(cluster=cluster{"starting address":u16, "values":u16[]} {"starting address"=0, "values"=[]}, "starting address"=w283, "values"=w279) -> (w285:cluster{"starting address":u16, "values":u16[]})
        n239 = Enqueue Element(queue=w284, element=w285) -> ()  [unwired: 2 in, 3 out]
      }
      event "启动": Mouse Down {
        n240 = event-data() -> ()  [unwired: 1 in, 8 out]
        n241 = flat-sequence {
          tunnel: w317 -> [w320]
          tunnel: [w320] -> w316
          tunnel: [w319] -> w313
          tunnel: w316 -> [w323]
          tunnel: [w323] -> w315
          tunnel: [w321] -> w314
          tunnel: w313 -> [w321]
          tunnel: w315 -> [w325]
          tunnel: w314 -> [w324]
          frame #0 {
            n242 = call "启动测量模式选择对话框.vi"() -> ("启动选择 2"=w319:u16)  [unwired: 11 in]
            "启动选择 2" <- w319
          }
          frame #1 {
            n243 = property on="启动选择 2" class="Ring (严格)"() -> ("RingText.Text"=w322:string)  [unwired: 2 in, 2 out]
            n244 = global write "COD测量模式全局.vi" "测量模式"(w322) -> ()
          }
          frame #2 {
            n245 = case shown="9, 默认" w324 {
              tunnel: [u16 4608 ("address") u16 4608 ("address") u16 4608 ("address") u16 4608 ("address") u16 4608 ("address") u16 4608 ("address") u16 4608 ("address") u16 4608 ("address") u16 4608 ("address") u16 4608 ("address")] -> w326
              tunnel: [u16 1 ("address") u16 2 ("address") u16 3 ("address") u16 4 ("address") u16 5 ("address") u16 7 ("address") u16 6 ("address") u16 8 ("address") u16 9 ("address") u16 0 ("address")] -> w327
              frame 0 {
              }
              frame 1 {
              }
              frame 2 {
              }
              frame 3 {
              }
              frame 4 {
              }
              frame 5 {
              }
              frame 6 {
              }
              frame 7 {
              }
              frame 8 {
              }
              frame 9, Default {
              }
            }
            n246 = Insert Into Array(array=u16[] [] ("values"), index=0 ("索引"), new element=w327) -> (w332:u16[])
            n247 = Bundle By Name(cluster=cluster{"starting address":u16, "values":u16[]} {"starting address"=0, "values"=[]}, "starting address"=w326, "values"=w332) -> (w329:cluster{"starting address":u16, "values":u16[]})
            n248 = Enqueue Element(queue=w325, element=w329) -> ()  [unwired: 2 in, 3 out]
          }
        }
        n249 = local write "枚举"(enum16{"读取数据", "写入数据", "读取写入DATABASE", "读取参数"}."写入数据" ("枚举")) -> ()
      }
      event "停止": Value Change {
        n250 = event-data() -> ()  [unwired: 1 in, 6 out]
        n251 = local write "枚举"(enum16{"读取数据", "写入数据", "读取写入DATABASE", "读取参数"}."写入数据" ("枚举")) -> ()
        n252 = Bundle By Name(cluster=cluster{"starting address":u16, "values":u16[]} {"starting address"=0, "values"=[]}, "starting address"=u16 4608, "values"=u16[] [11]) -> (w356:cluster{"starting address":u16, "values":u16[]})
        n253 = Enqueue Element(queue=w354, element=w356) -> ()  [unwired: 2 in, 3 out]
      }
      event "手动控制": Value Change {
        n254 = event-data() -> ()  [unwired: 1 in, 6 out]
        n255 = call "数字密码键盘.vi"() -> ("NewNumber"=w361:sgl)  [unwired: 1 in]
        n256 = Equal?(x=w361, y=8.0) -> (x = y?=w362:bool)
        n257 = case shown="真" w362 {
          tunnel: w360 -> [_ w366]
          tunnel: w359 -> [_ w365]
          frame False {
            n258 = call "窗口弹出对话框(子VI).vi"("消息"="密码错误") -> ()  [unwired: 10 in, 1 out]
          }
          frame True {
            n259 = call "CODMn手动控制框.vi"("Error in"=w365, "MB_Serial session"=w366) -> ()  [unwired: 10 in]
          }
        }
      }
      event "参数配置": Value Change {
        w374 = "CODMn是否切换量程" ("key")
        n260 = event-data() -> ()  [unwired: 1 in, 6 out]
        n261 = property on="窗格" class="Pane"("Origin"=T9 {"Horizontal"=0, "Vertical"=650} ("原点")) -> ()  [unwired: 2 in, 2 out]
        n262 = Bundle By Name(cluster=T5 {"starting address"=0, "number of holding registers"=0}, "starting address"=u16 4240, "number of holding registers"=u16 16) -> (w394:T5)
        n263 = local write "读取KB值"(FALSE ("读取KB值")) -> ()
        n264 = local write "枚举"(enum16{"读取数据", "写入数据", "读取写入DATABASE", "读取参数"}."读取参数" ("枚举")) -> ()
        n265 = Flush Queue(queue=w387, error in (no error)=w386) -> (queue out=w390:refnum<queue>, error out=w389:errorcluster)  [unwired: 1 out]
        n266 = Enqueue Element(queue=w390, element=w394, error in (no error)=w389) -> ()  [unwired: 1 in, 3 out]
        n267 = call <vilib>:"Application Directory.vi"() -> ("Application Directory"=w382:path)
        n268 = Build Path(base path=w382, name or relative path="data\\Set.ini" ("名称或相对路径")) -> (appended path=w380:path)
        n269 = call <vilib>:"Open Config Data.vi"("configuration file path"=w380) -> ("error out"=w383:errorcluster, "refnum"=w384:T10)  [unwired: 8 in, 1 out]
        n270 = call-poly <vilib>:"Read Key.vi"("section"=w374, "error in (no error)"=w383, "key"="自动切换量程", "refnum"=w384) -> ("error out"=w377:errorcluster, "value"=w367:u32, "refnum out"=w378:T10)  [unwired: 4 in, 1 out]
        n271 = local write "自动切换量程"(w367) -> ()
        n272 = call-poly <vilib>:"Read Key.vi"("section"=w374, "error in (no error)"=w377, "key"="低切高阈值", "refnum"=w378) -> ("error out"=w375:errorcluster, "value"=w369:dbl, "refnum out"=w376:T10)  [unwired: 4 in, 1 out]
        n273 = local write "低切高阈值"(w369) -> ()
        n274 = call-poly <vilib>:"Read Key.vi"("section"=w374, "error in (no error)"=w375, "key"="高切低阈值", "refnum"=w376) -> ("error out"=w372:errorcluster, "value"=w368:dbl, "refnum out"=w373:T10)  [unwired: 4 in, 1 out]
        n275 = local write "高切低阈值"(w368) -> ()
        n276 = call <vilib>:"Close Config Data.vi"("error in (no error)"=w372, "refnum"=w373) -> ()  [unwired: 8 in, 2 out]
      }
      event "保存": Mouse Down {
        n277 = event-data() -> ()  [unwired: 1 in, 8 out]
        n278 = call <vilib>:"Application Directory.vi"() -> ("Application Directory"=w422:path)
        n279 = Build Path(base path=w422, name or relative path="data\\Set.ini" ("名称或相对路径")) -> (appended path=w424:path)
        n280 = local write "枚举"(enum16{"读取数据", "写入数据", "读取写入DATABASE", "读取参数"}."写入数据" ("枚举")) -> ()
        n281 = local read "跨度液浓度"() -> (w419:dbl)
        n282 = call <vilib>:"Open Config Data.vi"("configuration file path"=w424) -> ("error out"=w426:errorcluster, "refnum"=w425:T10)  [unwired: 8 in, 1 out]
        n283 = call-poly <vilib>:"Write Key.vi"("section"="CODMn参数" ("key"), "error in (no error)"=w426, "value"=w419, "key"="跨度液浓度", "refnum"=w425) -> ("error out"=w428:errorcluster, "refnum out"=w427:T10)  [unwired: 4 in, 1 out]
        n284 = call <vilib>:"Close Config Data.vi"("error in (no error)"=w428, "refnum"=w427) -> ()  [unwired: 8 in, 2 out]
        n285 = local write "水样"("水样") -> ()
        n286 = local write "标液"("标液") -> ()
        n287 = local write "硫酸"("硫酸") -> ()
        n288 = local write "恒温时间"("恒温时间") -> ()
        n289 = local write "修正系数"("修正系数") -> ()
        n290 = local write "加标回收"("加标回收") -> ()
        n291 = local write "高锰酸钾"("高锰酸钾") -> ()
        n292 = local write "基本量程"("基本量程") -> ()
        n293 = local write "标样浓度 2"("标样浓度 2") -> ()
        n294 = local write "零点泵计量数 2"("零点泵计量数 2") -> ()
        n295 = local write "标度泵计量数 2"("标度泵计量数 2") -> ()
        n296 = local write "温度 2"("温度 2") -> ()
        n297 = local write "蒸馏水"("蒸馏水") -> ()
        n298 = local write "草酸钠"("草酸钠") -> ()
        n299 = local write "质控样"("质控样") -> ()
        n300 = Build Array("温度 2", "恒温时间", "浓度", "修正系数", "基本量程", "水样", "蒸馏水", "标液", "质控样", "加标回收", "高锰酸钾", "草酸钠", "硫酸", "零点泵计量数 2", "标度泵计量数 2", "标样浓度 2") -> (w411:dbl[])
        n301 = Bundle By Name(cluster=cluster{"starting address":u16, "values":u16[]} {"starting address"=4272, "values"=[]}, "starting address"=u16 4272, "values"=w411) -> (w413:cluster{"starting address":u16, "values":u16[]})
        n302 = Enqueue Element(queue=w396, element=w413, timeout in ms (-1)=1000 ("超时毫秒(-1)")) -> ()  [unwired: 1 in, 3 out]
      }
      event "校准配置": Value Change {
        n303 = event-data() -> ()  [unwired: 1 in, 6 out]
        n304 = property on="窗格" class="Pane"("Origin"=T9 {"Horizontal"=0, "Vertical"=1300} ("原点")) -> ()  [unwired: 2 in, 2 out]
        n305 = call <vilib>:"Application Directory.vi"() -> ("Application Directory"=w479:path)
        n306 = Build Path(base path=w479, name or relative path="data\\Set.ini" ("名称或相对路径")) -> (appended path=w477:path)
        n307 = call <vilib>:"Open Config Data.vi"("configuration file path"=w477) -> ("error out"=w447:errorcluster, "refnum"=w448:T10)  [unwired: 8 in, 1 out]
        n308 = call-poly <vilib>:"Read Key.vi"("section"="CODMn模型选择" ("key"), "error in (no error)"=w447, "key"="线性和多项式", "refnum"=w448) -> ("error out"=w443:errorcluster, "value"=w446:i32, "refnum out"=w444:T10)  [unwired: 4 in, 1 out]
        n309 = local write "模型"(w446) -> ()
        n310 = call-poly <vilib>:"Read Key.vi"("section"="标线选择", "error in (no error)"=w443, "key"="选用水样", "refnum"=w444) -> ("error out"=w441:errorcluster, "value"=w445:i32, "refnum out"=w442:T10)  [unwired: 4 in, 1 out]
        n311 = local write "选用水样"(w445) -> ()
        n312 = local read "量程选择"() -> (w454:enum16{"低量程", "高量程", "0-2量程"})
        n313 = case shown="0, 默认" w445 {
          tunnel: ["葡萄糖标线" ("section") "草酸钠标线" ("section")] -> w453
          frame 0, Default {
          }
          frame 1 {
          }
        }
        n314 = case shown="\"0-2量程\"" w454 {
          tunnel: ["低量程" "高量程" "0-2量程"] -> w452
          frame "低量程", Default {
          }
          frame "高量程" {
          }
          frame "0-2量程" {
          }
        }
        n315 = Concatenate Strings(w453, w452) -> (w451:string)
        n316 = call-poly <vilib>:"Read Key.vi"("section"=w451, "error in (no error)"=w441, "key"="浓度1", "refnum"=w442) -> ("error out"=w483:errorcluster, "value"=w481:dbl, "refnum out"=w482:T10)  [unwired: 4 in, 1 out]
        n317 = local write "浓度1"(w481) -> ()
        n318 = call-poly <vilib>:"Read Key.vi"("section"=w451, "error in (no error)"=w483, "key"="浓度2", "refnum"=w482) -> ("error out"=w497:errorcluster, "value"=w484:dbl, "refnum out"=w496:T10)  [unwired: 4 in, 1 out]
        n319 = local write "浓度2"(w484) -> ()
        n320 = call-poly <vilib>:"Read Key.vi"("section"=w451, "error in (no error)"=w497, "key"="浓度3", "refnum"=w496) -> ("error out"=w498:errorcluster, "value"=w486:dbl, "refnum out"=w495:T10)  [unwired: 4 in, 1 out]
        n321 = local write "浓度3"(w486) -> ()
        n322 = call-poly <vilib>:"Read Key.vi"("section"=w451, "error in (no error)"=w498, "key"="泵滴定数1", "refnum"=w495) -> ("error out"=w499:errorcluster, "value"=w488:dbl, "refnum out"=w494:T10)  [unwired: 4 in, 1 out]
        n323 = local write "泵滴定数1"(w488) -> ()
        n324 = call-poly <vilib>:"Read Key.vi"("section"=w451, "error in (no error)"=w499, "key"="泵滴定数2", "refnum"=w494) -> ("error out"=w493:errorcluster, "value"=w491:dbl, "refnum out"=w500:T10)  [unwired: 4 in, 1 out]
        n325 = local write "泵滴定数2"(w491) -> ()
        n326 = call-poly <vilib>:"Read Key.vi"("section"=w451, "error in (no error)"=w493, "key"="泵滴定数3", "refnum"=w500) -> ("error out"=w505:errorcluster, "value"=w504:dbl, "refnum out"=w501:T10)  [unwired: 4 in, 1 out]
        n327 = local write "泵滴定数3"(w504) -> ()
        n328 = call-poly <vilib>:"Read Key.vi"("section"=w451, "error in (no error)"=w505, "key"="浓度4", "refnum"=w501) -> ("error out"=w506:errorcluster, "value"=w434:dbl, "refnum out"=w502:T10)  [unwired: 4 in, 1 out]
        n329 = local write "浓度4"(w434) -> ()
        n330 = call-poly <vilib>:"Read Key.vi"("section"=w451, "error in (no error)"=w506, "key"="浓度5", "refnum"=w502) -> ("error out"=w439:errorcluster, "value"=w433:dbl, "refnum out"=w440:T10)  [unwired: 4 in, 1 out]
        n331 = local write "浓度5"(w433) -> ()
        n332 = call-poly <vilib>:"Read Key.vi"("section"=w451, "error in (no error)"=w439, "key"="泵滴定数4", "refnum"=w440) -> ("error out"=w507:errorcluster, "value"=w432:dbl, "refnum out"=w503:T10)  [unwired: 4 in, 1 out]
        n333 = local write "泵滴定数4"(w432) -> ()
        n334 = call-poly <vilib>:"Read Key.vi"("section"=w451, "error in (no error)"=w507, "key"="泵滴定数5", "refnum"=w503) -> ("error out"=w437:errorcluster, "value"=w431:dbl, "refnum out"=w438:T10)  [unwired: 4 in, 1 out]
        n335 = local write "泵滴定数5"(w431) -> ()
        n336 = call-poly <vilib>:"Read Key.vi"("section"=w451, "error in (no error)"=w437, "key"="当前选用的校准", "refnum"=w438) -> ("error out"=w473:errorcluster, "value"=w475:i32, "refnum out"=w474:T10)  [unwired: 4 in, 1 out]
        n337 = local write "当前校准"(w475) -> ()
        n338 = call-poly <vilib>:"Read Key.vi"("section"=w451, "error in (no error)"=w473, "key"="启用1", "refnum"=w474) -> ("error out"=w470:errorcluster, "value"=w459:bool, "refnum out"=w471:T10)  [unwired: 4 in, 1 out]
        n339 = local write "启用1"(w459) -> ()
        n340 = call-poly <vilib>:"Read Key.vi"("section"=w451, "error in (no error)"=w470, "key"="启用2", "refnum"=w471) -> ("error out"=w468:errorcluster, "value"=w458:bool, "refnum out"=w469:T10)  [unwired: 4 in, 1 out]
        n341 = local write "启用2"(w458) -> ()
        n342 = call-poly <vilib>:"Read Key.vi"("section"=w451, "error in (no error)"=w468, "key"="启用3", "refnum"=w469) -> ("error out"=w466:errorcluster, "value"=w457:bool, "refnum out"=w467:T10)  [unwired: 4 in, 1 out]
        n343 = local write "启用3"(w457) -> ()
        n344 = call-poly <vilib>:"Read Key.vi"("section"=w451, "error in (no error)"=w466, "key"="启用4", "refnum"=w467) -> ("error out"=w464:errorcluster, "value"=w430:bool, "refnum out"=w465:T10)  [unwired: 4 in, 1 out]
        n345 = local write "启用4"(w430) -> ()
        n346 = call-poly <vilib>:"Read Key.vi"("section"=w451, "error in (no error)"=w464, "key"="启用5", "refnum"=w465) -> ("error out"=w435:errorcluster, "value"=w429:bool, "refnum out"=w436:T10)  [unwired: 4 in, 1 out]
        n347 = local write "启用5"(w429) -> ()
        n348 = call <vilib>:"Close Config Data.vi"("error in (no error)"=w435, "refnum"=w436) -> ()  [unwired: 8 in, 2 out]
      }
      event "选用水样": Value Change {
        (unwired) "浓度6" ("key")
        n349 = event-data() -> ()  [unwired: 1 in, 6 out]
        n350 = property on="窗格" class="Pane"("Origin"=T9 {"Horizontal"=0, "Vertical"=1300} ("原点")) -> ()  [unwired: 2 in, 2 out]
        n351 = local read "量程选择"() -> (w531:enum16{"低量程", "高量程", "0-2量程"})
        n352 = case shown="\"0-2量程\"" w531 {
          tunnel: ["低量程" "高量程" "0-2量程"] -> w532
          frame "低量程", Default {
          }
          frame "高量程" {
          }
          frame "0-2量程" {
          }
        }
        n353 = case shown="\"葡萄糖\", 默认" "选用水样" {
          tunnel: ["葡萄糖标线" ("section") "草酸钠标线" ("section")] -> w533
          frame "葡萄糖", Default {
          }
          frame "草酸钠" {
          }
        }
        n354 = call <vilib>:"Application Directory.vi"() -> ("Application Directory"=w557:path)
        n355 = Build Path(base path=w557, name or relative path="data\\Set.ini" ("名称或相对路径")) -> (appended path=w555:path)
        n356 = call <vilib>:"Open Config Data.vi"("configuration file path"=w555) -> ("error out"=w558:errorcluster, "refnum"=w559:T10)  [unwired: 8 in, 1 out]
        n357 = Concatenate Strings(w533, w532) -> (w530:string)
        n358 = call-poly <vilib>:"Read Key.vi"("section"=w530, "error in (no error)"=w558, "key"="浓度1", "refnum"=w559) -> ("error out"=w563:errorcluster, "value"=w561:dbl, "refnum out"=w562:T10)  [unwired: 4 in, 1 out]
        n359 = local write "浓度1"(w561) -> ()
        n360 = call-poly <vilib>:"Read Key.vi"("section"=w530, "error in (no error)"=w563, "key"="浓度2", "refnum"=w562) -> ("error out"=w577:errorcluster, "value"=w564:dbl, "refnum out"=w576:T10)  [unwired: 4 in, 1 out]
        n361 = local write "浓度2"(w564) -> ()
        n362 = call-poly <vilib>:"Read Key.vi"("section"=w530, "error in (no error)"=w577, "key"="浓度3", "refnum"=w576) -> ("error out"=w578:errorcluster, "value"=w566:dbl, "refnum out"=w575:T10)  [unwired: 4 in, 1 out]
        n363 = local write "浓度3"(w566) -> ()
        n364 = call-poly <vilib>:"Read Key.vi"("section"=w530, "error in (no error)"=w578, "key"="泵滴定数1", "refnum"=w575) -> ("error out"=w579:errorcluster, "value"=w568:dbl, "refnum out"=w574:T10)  [unwired: 4 in, 1 out]
        n365 = local write "泵滴定数1"(w568) -> ()
        n366 = call-poly <vilib>:"Read Key.vi"("section"=w530, "error in (no error)"=w579, "key"="泵滴定数2", "refnum"=w574) -> ("error out"=w573:errorcluster, "value"=w571:dbl, "refnum out"=w580:T10)  [unwired: 4 in, 1 out]
        n367 = local write "泵滴定数2"(w571) -> ()
        n368 = call-poly <vilib>:"Read Key.vi"("section"=w530, "error in (no error)"=w573, "key"="泵滴定数3", "refnum"=w580) -> ("error out"=w585:errorcluster, "value"=w584:dbl, "refnum out"=w581:T10)  [unwired: 4 in, 1 out]
        n369 = local write "泵滴定数3"(w584) -> ()
        n370 = call-poly <vilib>:"Read Key.vi"("section"=w530, "error in (no error)"=w585, "key"="浓度4", "refnum"=w581) -> ("error out"=w586:errorcluster, "value"=w525:dbl, "refnum out"=w582:T10)  [unwired: 4 in, 1 out]
        n371 = local write "浓度4"(w525) -> ()
        n372 = call-poly <vilib>:"Read Key.vi"("section"=w530, "error in (no error)"=w586, "key"="浓度5", "refnum"=w582) -> ("error out"=w528:errorcluster, "value"=w524:dbl, "refnum out"=w529:T10)  [unwired: 4 in, 1 out]
        n373 = local write "浓度5"(w524) -> ()
        n374 = call-poly <vilib>:"Read Key.vi"("section"=w530, "error in (no error)"=w528, "key"="泵滴定数4", "refnum"=w529) -> ("error out"=w587:errorcluster, "value"=w523:dbl, "refnum out"=w583:T10)  [unwired: 4 in, 1 out]
        n375 = local write "泵滴定数4"(w523) -> ()
        n376 = call-poly <vilib>:"Read Key.vi"("section"=w530, "error in (no error)"=w587, "key"="泵滴定数5", "refnum"=w583) -> ("error out"=w526:errorcluster, "value"=w522:dbl, "refnum out"=w527:T10)  [unwired: 4 in, 1 out]
        n377 = local write "泵滴定数5"(w522) -> ()
        n378 = call-poly <vilib>:"Read Key.vi"("section"=w530, "error in (no error)"=w526, "key"="当前选用的校准", "refnum"=w527) -> ("error out"=w551:errorcluster, "value"=w553:i32, "refnum out"=w552:T10)  [unwired: 4 in, 1 out]
        n379 = local write "当前校准"(w553) -> ()
        n380 = call-poly <vilib>:"Read Key.vi"("section"=w530, "error in (no error)"=w551, "key"="启用1", "refnum"=w552) -> ("error out"=w548:errorcluster, "value"=w537:bool, "refnum out"=w549:T10)  [unwired: 4 in, 1 out]
        n381 = local write "启用1"(w537) -> ()
        n382 = call-poly <vilib>:"Read Key.vi"("section"=w530, "error in (no error)"=w548, "key"="启用2", "refnum"=w549) -> ("error out"=w546:errorcluster, "value"=w536:bool, "refnum out"=w547:T10)  [unwired: 4 in, 1 out]
        n383 = local write "启用2"(w536) -> ()
        n384 = call-poly <vilib>:"Read Key.vi"("section"=w530, "error in (no error)"=w546, "key"="启用3", "refnum"=w547) -> ("error out"=w544:errorcluster, "value"=w535:bool, "refnum out"=w545:T10)  [unwired: 4 in, 1 out]
        n385 = local write "启用3"(w535) -> ()
        n386 = call-poly <vilib>:"Read Key.vi"("section"=w530, "error in (no error)"=w544, "key"="启用4", "refnum"=w545) -> ("error out"=w542:errorcluster, "value"=w519:bool, "refnum out"=w543:T10)  [unwired: 4 in, 1 out]
        n387 = local write "启用4"(w519) -> ()
        n388 = call-poly <vilib>:"Read Key.vi"("section"=w530, "error in (no error)"=w542, "key"="启用5", "refnum"=w543) -> ("error out"=w520:errorcluster, "value"=w518:bool, "refnum out"=w521:T10)  [unwired: 4 in, 1 out]
        n389 = local write "启用5"(w518) -> ()
        n390 = call <vilib>:"Close Config Data.vi"("error in (no error)"=w520, "refnum"=w521) -> ()  [unwired: 8 in, 2 out]
      }
      event "量程选择": Value Change {
        n391 = event-data() -> ()  [unwired: 1 in, 6 out]
        n392 = property on="窗格" class="Pane"("Origin"=T9 {"Horizontal"=0, "Vertical"=1300} ("原点")) -> ()  [unwired: 2 in, 2 out]
        n393 = local read "选用水样"() -> (w614:enum16{"葡萄糖", "草酸钠"})
        n394 = case shown="\"葡萄糖\", 默认" w614 {
          tunnel: ["葡萄糖标线" ("section") "草酸钠标线" ("section")] -> w613
          frame "葡萄糖", Default {
          }
          frame "草酸钠" {
          }
        }
        n395 = case shown="\"0-2量程\"" "量程选择" {
          tunnel: ["低量程" "高量程" "0-2量程"] -> w610
          frame "低量程", Default {
          }
          frame "高量程" {
          }
          frame "0-2量程" {
          }
        }
        n396 = call <vilib>:"Application Directory.vi"() -> ("Application Directory"=w637:path)
        n397 = Build Path(base path=w637, name or relative path="data\\Set.ini" ("名称或相对路径")) -> (appended path=w635:path)
        n398 = call <vilib>:"Open Config Data.vi"("configuration file path"=w635) -> ("error out"=w638:errorcluster, "refnum"=w639:T10)  [unwired: 8 in, 1 out]
        n399 = Concatenate Strings(w613, w610) -> (w612:string)
        n400 = call-poly <vilib>:"Read Key.vi"("section"=w612, "error in (no error)"=w638, "key"="浓度1", "refnum"=w639) -> ("error out"=w643:errorcluster, "value"=w641:dbl, "refnum out"=w642:T10)  [unwired: 4 in, 1 out]
        n401 = local write "浓度1"(w641) -> ()
        n402 = call-poly <vilib>:"Read Key.vi"("section"=w612, "error in (no error)"=w643, "key"="浓度2", "refnum"=w642) -> ("error out"=w657:errorcluster, "value"=w644:dbl, "refnum out"=w656:T10)  [unwired: 4 in, 1 out]
        n403 = local write "浓度2"(w644) -> ()
        n404 = call-poly <vilib>:"Read Key.vi"("section"=w612, "error in (no error)"=w657, "key"="浓度3", "refnum"=w656) -> ("error out"=w658:errorcluster, "value"=w646:dbl, "refnum out"=w655:T10)  [unwired: 4 in, 1 out]
        n405 = local write "浓度3"(w646) -> ()
        n406 = call-poly <vilib>:"Read Key.vi"("section"=w612, "error in (no error)"=w658, "key"="泵滴定数1", "refnum"=w655) -> ("error out"=w659:errorcluster, "value"=w648:dbl, "refnum out"=w654:T10)  [unwired: 4 in, 1 out]
        n407 = local write "泵滴定数1"(w648) -> ()
        n408 = call-poly <vilib>:"Read Key.vi"("section"=w612, "error in (no error)"=w659, "key"="泵滴定数2", "refnum"=w654) -> ("error out"=w653:errorcluster, "value"=w651:dbl, "refnum out"=w660:T10)  [unwired: 4 in, 1 out]
        n409 = local write "泵滴定数2"(w651) -> ()
        n410 = call-poly <vilib>:"Read Key.vi"("section"=w612, "error in (no error)"=w653, "key"="泵滴定数3", "refnum"=w660) -> ("error out"=w665:errorcluster, "value"=w664:dbl, "refnum out"=w661:T10)  [unwired: 4 in, 1 out]
        n411 = local write "泵滴定数3"(w664) -> ()
        n412 = call-poly <vilib>:"Read Key.vi"("section"=w612, "error in (no error)"=w665, "key"="浓度4", "refnum"=w661) -> ("error out"=w666:errorcluster, "value"=w601:dbl, "refnum out"=w662:T10)  [unwired: 4 in, 1 out]
        n413 = local write "浓度4"(w601) -> ()
        n414 = call-poly <vilib>:"Read Key.vi"("section"=w612, "error in (no error)"=w666, "key"="浓度5", "refnum"=w662) -> ("error out"=w608:errorcluster, "value"=w600:dbl, "refnum out"=w609:T10)  [unwired: 4 in, 1 out]
        n415 = local write "浓度5"(w600) -> ()
        n416 = call-poly <vilib>:"Read Key.vi"("section"=w612, "error in (no error)"=w608, "key"="泵滴定数4", "refnum"=w609) -> ("error out"=w667:errorcluster, "value"=w599:dbl, "refnum out"=w663:T10)  [unwired: 4 in, 1 out]
        n417 = local write "泵滴定数4"(w599) -> ()
        n418 = call-poly <vilib>:"Read Key.vi"("section"=w612, "error in (no error)"=w667, "key"="泵滴定数5", "refnum"=w663) -> ("error out"=w606:errorcluster, "value"=w598:dbl, "refnum out"=w607:T10)  [unwired: 4 in, 1 out]
        n419 = local write "泵滴定数5"(w598) -> ()
        n420 = call-poly <vilib>:"Read Key.vi"("section"=w612, "error in (no error)"=w606, "key"="当前选用的校准", "refnum"=w607) -> ("error out"=w631:errorcluster, "value"=w633:i32, "refnum out"=w632:T10)  [unwired: 4 in, 1 out]
        n421 = local write "当前校准"(w633) -> ()
        n422 = call-poly <vilib>:"Read Key.vi"("section"=w612, "error in (no error)"=w631, "key"="启用1", "refnum"=w632) -> ("error out"=w628:errorcluster, "value"=w617:bool, "refnum out"=w629:T10)  [unwired: 4 in, 1 out]
        n423 = local write "启用1"(w617) -> ()
        n424 = call-poly <vilib>:"Read Key.vi"("section"=w612, "error in (no error)"=w628, "key"="启用2", "refnum"=w629) -> ("error out"=w626:errorcluster, "value"=w616:bool, "refnum out"=w627:T10)  [unwired: 4 in, 1 out]
        n425 = local write "启用2"(w616) -> ()
        n426 = call-poly <vilib>:"Read Key.vi"("section"=w612, "error in (no error)"=w626, "key"="启用3", "refnum"=w627) -> ("error out"=w624:errorcluster, "value"=w615:bool, "refnum out"=w625:T10)  [unwired: 4 in, 1 out]
        n427 = local write "启用3"(w615) -> ()
        n428 = call-poly <vilib>:"Read Key.vi"("section"=w612, "error in (no error)"=w624, "key"="启用4", "refnum"=w625) -> ("error out"=w622:errorcluster, "value"=w603:bool, "refnum out"=w623:T10)  [unwired: 4 in, 1 out]
        n429 = local write "启用4"(w603) -> ()
        n430 = call-poly <vilib>:"Read Key.vi"("section"=w612, "error in (no error)"=w622, "key"="启用5", "refnum"=w623) -> ("error out"=w604:errorcluster, "value"=w602:bool, "refnum out"=w605:T10)  [unwired: 4 in, 1 out]
        n431 = local write "启用5"(w602) -> ()
        n432 = call <vilib>:"Close Config Data.vi"("error in (no error)"=w604, "refnum"=w605) -> ()  [unwired: 8 in, 2 out]
      }
      event "周期设置": Value Change {
        n433 = event-data() -> ()  [unwired: 1 in, 6 out]
        n434 = call "数字密码键盘.vi"() -> ("NewNumber"=w678:sgl)  [unwired: 1 in]
        n435 = Equal?(x=w678, y=8.0) -> (x = y?=w679:bool)
        n436 = case shown="真" w679 {
          frame False {
            n437 = call "窗口弹出对话框(子VI).vi"("消息"="密码错误") -> ()  [unwired: 10 in, 1 out]
          }
          frame True {
            n438 = call "窗口弹出对话框(子VI).vi"("消息"="登录成功") -> ("true"=w682:bool)  [unwired: 10 in]
            n439 = case shown="真" w682 {
              frame False {
              }
              frame True {
                n440 = property on="窗格" class="Pane"("Origin"=T9 {"Horizontal"=0, "Vertical"=1950} ("原点")) -> ()  [unwired: 2 in, 2 out]
              }
            }
          }
        }
      }
      event "返回": Value Change {
        (unwired) "泵滴定数6" ("key")
        w698 = "CODMn" ("section")
        n441 = event-data() -> ()  [unwired: 1 in, 6 out]
        n442 = property on="窗格" class="Pane"("Origin"=T9 {"Horizontal"=0, "Vertical"=0} ("原点")) -> ()  [unwired: 2 in, 2 out]
        n443 = call <vilib>:"Application Directory.vi"() -> ("Application Directory"=w751:path)
        n444 = Build Path(base path=w751, name or relative path="data\\Set.ini" ("名称或相对路径")) -> (appended path=w749:path)
        n445 = local write "读取KB值"(FALSE ("读取KB值")) -> ()
        n446 = call <vilib>:"Open Config Data.vi"("configuration file path"=w749) -> ("error out"=w747:errorcluster, "refnum"=w748:T10)  [unwired: 8 in, 1 out]
        n447 = local read "浓度1"() -> (w745:dbl)
        n448 = local read "浓度2"() -> (w729:dbl)
        n449 = call-poly <vilib>:"Write Key.vi"("section"=w698, "error in (no error)"=w747, "value"=w745, "key"="浓度1", "refnum"=w748) -> ("error out"=w744:errorcluster, "refnum out"=w743:T10)  [unwired: 4 in, 1 out]
        n450 = local read "浓度3"() -> (w725:dbl)
        n451 = call-poly <vilib>:"Write Key.vi"("section"=w698, "error in (no error)"=w744, "value"=w729, "key"="浓度2", "refnum"=w743) -> ("error out"=w742:errorcluster, "refnum out"=w741:T10)  [unwired: 4 in, 1 out]
        n452 = local read "泵滴定数1"() -> (w723:dbl)
        n453 = call-poly <vilib>:"Write Key.vi"("section"=w698, "error in (no error)"=w742, "value"=w725, "key"="浓度3", "refnum"=w741) -> ("error out"=w740:errorcluster, "refnum out"=w739:T10)  [unwired: 4 in, 1 out]
        n454 = call-poly <vilib>:"Write Key.vi"("section"=w698, "error in (no error)"=w740, "value"=w723, "key"="泵滴定数1", "refnum"=w739) -> ("error out"=w738:errorcluster, "refnum out"=w737:T10)  [unwired: 4 in, 1 out]
        n455 = local read "泵滴定数2"() -> (w721:dbl)
        n456 = call-poly <vilib>:"Write Key.vi"("section"=w698, "error in (no error)"=w738, "value"=w721, "key"="泵滴定数2", "refnum"=w737) -> ("error out"=w736:errorcluster, "refnum out"=w735:T10)  [unwired: 4 in, 1 out]
        n457 = local read "泵滴定数3"() -> (w719:dbl)
        n458 = local read "浓度4"() -> (w686:dbl)
        n459 = call-poly <vilib>:"Write Key.vi"("section"=w698, "error in (no error)"=w736, "value"=w719, "key"="泵滴定数3", "refnum"=w735) -> ("error out"=w734:errorcluster, "refnum out"=w733:T10)  [unwired: 4 in, 1 out]
        n460 = call-poly <vilib>:"Write Key.vi"("section"=w698, "error in (no error)"=w734, "value"=w686, "key"="浓度4", "refnum"=w733) -> ("error out"=w727:errorcluster, "refnum out"=w728:T10)  [unwired: 4 in, 1 out]
        n461 = local read "浓度5"() -> (w685:dbl)
        n462 = call-poly <vilib>:"Write Key.vi"("section"=w698, "error in (no error)"=w727, "value"=w685, "key"="浓度5", "refnum"=w728) -> ("error out"=w695:errorcluster, "refnum out"=w696:T10)  [unwired: 4 in, 1 out]
        n463 = local read "泵滴定数4"() -> (w687:dbl)
        n464 = call-poly <vilib>:"Write Key.vi"("section"=w698, "error in (no error)"=w695, "value"=w687, "key"="泵滴定数4", "refnum"=w696) -> ("error out"=w732:errorcluster, "refnum out"=w731:T10)  [unwired: 4 in, 1 out]
        n465 = local read "泵滴定数5"() -> (w688:dbl)
        n466 = call-poly <vilib>:"Write Key.vi"("section"=w698, "error in (no error)"=w732, "value"=w688, "key"="泵滴定数5", "refnum"=w731) -> ("error out"=w693:errorcluster, "refnum out"=w694:T10)  [unwired: 4 in, 1 out]
        n467 = local read "启用1"() -> (w707:bool)
        n468 = call-poly <vilib>:"Write Key.vi"("section"=w698, "error in (no error)"=w693, "value"=w707, "key"="启用1", "refnum"=w694) -> ("error out"=w703:errorcluster, "refnum out"=w706:T10)  [unwired: 4 in, 1 out]
        n469 = local read "启用2"() -> (w704:bool)
        n470 = call-poly <vilib>:"Write Key.vi"("section"=w698, "error in (no error)"=w703, "value"=w704, "key"="启用2", "refnum"=w706) -> ("error out"=w714:errorcluster, "refnum out"=w713:T10)  [unwired: 4 in, 1 out]
        n471 = local read "启用3"() -> (w702:bool)
        n472 = call-poly <vilib>:"Write Key.vi"("section"=w698, "error in (no error)"=w714, "value"=w702, "key"="启用3", "refnum"=w713) -> ("error out"=w712:errorcluster, "refnum out"=w711:T10)  [unwired: 4 in, 1 out]
        n473 = local read "启用4"() -> (w690:bool)
        n474 = call-poly <vilib>:"Write Key.vi"("section"=w698, "error in (no error)"=w712, "value"=w690, "key"="启用4", "refnum"=w711) -> ("error out"=w710:errorcluster, "refnum out"=w709:T10)  [unwired: 4 in, 1 out]
        n475 = local read "启用5"() -> (w689:bool)
        n476 = call-poly <vilib>:"Write Key.vi"("section"=w698, "error in (no error)"=w710, "value"=w689, "key"="启用5", "refnum"=w709) -> ("error out"=w691:errorcluster, "refnum out"=w692:T10)  [unwired: 4 in, 1 out]
        n477 = call <vilib>:"Close Config Data.vi"("error in (no error)"=w691, "refnum"=w692) -> ()  [unwired: 8 in, 2 out]
      }
      event "关闭", "关闭 2", "关闭 3": Value Change {
        n478 = event-data() -> ()  [unwired: 1 in, 6 out]
        n479 = property on="窗格" class="Pane"("Origin"=T9 {"Horizontal"=0, "Vertical"=0} ("原点")) -> ()  [unwired: 2 in, 2 out]
      }
      event Timeout; Application Instance Close {
        n480 = event-data() -> ()  [unwired: 1 in, 3 out]
        n481 = call-dynamic "Close Session.vi"("error in (no error)"=w754, "MB_Serial session"=w755) -> ()  [unwired: 9 in, 1 out]
      }
      event "时间校准": Value Change {
        n482 = event-data() -> ()  [unwired: 1 in, 6 out]
        n483 = flat-sequence {
          tunnel: w756 -> [w761]
          frame #0 {
            n484 = Get Date/Time In Seconds() -> (seconds since 1Jan1904=w766:timestamp)
            n485 = Build Array(w766) -> (w765:timestamp[])
            n486 = call "DateToHex.vi"("DATE"=w765) -> ("数组"=w759:u16[])  [unwired: 10 in]
            n487 = Insert Into Array(array=u16[] [1] ("values"), index=1 ("索引"), new element=w759) -> (w757:u16[])
            n488 = Bundle By Name(cluster=cluster{"starting address":u16, "values":u16[]} {"starting address"=0, "values"=[]}, "starting address"=u16 4612, "values"=w757) -> (w762:cluster{"starting address":u16, "values":u16[]})
            n489 = Enqueue Element(queue=w761, element=w762) -> ()  [unwired: 2 in, 3 out]
          }
          frame #1 {
            n490 = local write "枚举"(enum16{"读取数据", "写入数据", "读取写入DATABASE", "读取参数"}."写入数据" ("枚举")) -> ()
          }
        }
      }
      event "故障清除": Value Change {
        n491 = event-data() -> ()  [unwired: 1 in, 6 out]
        n492 = local write "枚举"(enum16{"读取数据", "写入数据", "读取写入DATABASE", "读取参数"}."写入数据" ("枚举")) -> ()
        n493 = Bundle By Name(cluster=cluster{"starting address":u16, "values":u16[]} {"starting address"=0, "values"=[]}, "starting address"=u16 4611, "values"=u16[] [1]) -> (w771:cluster{"starting address":u16, "values":u16[]})
        n494 = Enqueue Element(queue=w770, element=w771) -> ()  [unwired: 2 in, 3 out]
      }
      event "定时启动": Mouse Down {
        n495 = event-data() -> ()  [unwired: 1 in, 8 out]
        n496 = flat-sequence {
          frame #0 {
            n497 = global read "CODMn断电保存全局变量.vi" "定时控制"() -> (w774:T7)
            n498 = call "周期设置.vi"("定时控制参数输入"=w774) -> ("定时控制参数输出"=w775:T7)  [unwired: 10 in]
            n499 = global write "CODMn断电保存全局变量.vi" "定时控制"(w775) -> ()
          }
          frame #1 {
            n500 = call <vilib>:"Application Directory.vi"() -> ("Application Directory"=w789:path)
            n501 = Build Path(base path=w789, name or relative path="data\\sys.ini" ("名称或相对路径")) -> (appended path=w787:path)
            n502 = call <vilib>:"Open Config Data.vi"("configuration file path"=w787) -> ("error out"=w783:errorcluster, "refnum"=w786:T10)  [unwired: 8 in, 1 out]
            n503 = vi-ref "斯坦道CODMn.lvlib:CODMn断电保存全局变量.vi"() -> (w785:refnum<vi>)
            n504 = call <userlib>:"Write Panel to INI__ogtk.vi"("error in (no error)"=w783, "VI ref"=w785, "refnum"=w786) -> ("error out"=w782:errorcluster, "refnum out"=w784:T10)  [unwired: 7 in]
            n505 = call <vilib>:"Close Config Data.vi"("error in (no error)"=w782, "refnum"=w784) -> ("error out"=w777:errorcluster, "file path"=w776:path)  [unwired: 8 in]
            n506 = Open/Create/Replace File(file path (use dialog)=w776, error in=w777) -> (refnum out=w780:refnum<file>, error out=w781:errorcluster)  [unwired: 4 in, 1 out]
            n507 = Flush File(refnum=w780, error in=w781) -> (refnum out=w779:refnum<file>, error out=w778:errorcluster)
            n508 = Close File(refnum=w779, error in=w778) -> ()  [unwired: 2 out]
          }
        }
      }
      event "CODMn空白测试选择": Value Change {
        n509 = event-data() -> ()  [unwired: 1 in, 6 out]
        n510 = flat-sequence {
          frame #0 {
            n511 = global write "CODMn断电保存全局变量.vi" "CODMn空白测试选择"("CODMn空白测试选择") -> ()
          }
          frame #1 {
            n512 = call <vilib>:"Application Directory.vi"() -> ("Application Directory"=w804:path)
            n513 = Build Path(base path=w804, name or relative path="data\\sys.ini" ("名称或相对路径")) -> (appended path=w802:path)
            n514 = call <vilib>:"Open Config Data.vi"("configuration file path"=w802) -> ("error out"=w798:errorcluster, "refnum"=w801:T10)  [unwired: 8 in, 1 out]
            n515 = vi-ref "斯坦道CODMn.lvlib:CODMn断电保存全局变量.vi"() -> (w800:refnum<vi>)
            n516 = call <userlib>:"Write Panel to INI__ogtk.vi"("error in (no error)"=w798, "VI ref"=w800, "refnum"=w801) -> ("error out"=w797:errorcluster, "refnum out"=w799:T10)  [unwired: 7 in]
            n517 = call <vilib>:"Close Config Data.vi"("error in (no error)"=w797, "refnum"=w799) -> ("error out"=w792:errorcluster, "file path"=w791:path)  [unwired: 8 in]
            n518 = Open/Create/Replace File(file path (use dialog)=w791, error in=w792) -> (refnum out=w795:refnum<file>, error out=w796:errorcluster)  [unwired: 4 in, 1 out]
            n519 = Flush File(refnum=w795, error in=w796) -> (refnum out=w794:refnum<file>, error out=w793:errorcluster)
            n520 = Close File(refnum=w794, error in=w793) -> ()  [unwired: 2 out]
          }
        }
      }
      event "校准1", "校准2", "校准3", "校准4", "校准5": Value Change {
        n521 = event-data() -> ()  [unwired: 1 in, 6 out]
        n522 = flat-sequence {
          tunnel: w807 -> [w812]
          tunnel: [w811] -> w806
          tunnel: [w810] -> w805
          tunnel: w806 -> [w845]
          tunnel: w805 -> [w844]
          frame #0 {
            n523 = Build Array("校准1", "校准2", "校准3", "校准4", "校准5") -> (w813:bool[])
            n524 = for {
              tunnel: w813 -> [w827] mode=indexing
              tunnel: w812 -> [w823]
              tunnel: [w819] -> w811
              tunnel: [w818] -> w810
              i -> [w817]
              n525 = case shown="4" w817 {
                tunnel: ["浓度1" "浓度2" "浓度3" "浓度4" "浓度5"] -> w822
                frame 0, Default {
                }
                frame 1 {
                }
                frame 2 {
                }
                frame 3 {
                }
                frame 4 {
                }
              }
              n526 = Multiply(x=w822, y=100.0) -> (x*y=w820:dbl)
              n527 = Insert Into Array(array=u16[] [] ("values"), index=0 ("索引"), new element=w820) -> (w824:u16[])
              n528 = case shown="真" w827 {
                tunnel: w824 -> [_ w839]
                tunnel: w823 -> [w833 w838]
                tunnel: [w833 w837] -> w819
                tunnel: [_ w836] -> w818
                tunnel: w817 -> [_ w835]
                frame False {
                }
                frame True {
                  n529 = Increment(x=w835) -> (x+1=→"当前校准":i32)
                  n530 = Bundle By Name(cluster=cluster{"starting address":u16, "values":u16[]} {"starting address"=4272, "values"=[]}, "starting address"=u16 4274, "values"=w839) -> (w841:cluster{"starting address":u16, "values":u16[]})
                  n531 = Enqueue Element(queue=w838, element=w841) -> (queue out=w837:refnum<queue>, error out=w836:errorcluster)  [unwired: 2 in, 1 out]
                }
              }
            }
          }
          frame #1 {
            n532 = local read "当前校准"() -> (w850:i32)
            n533 = case shown="5" w850 {
              tunnel: [w856 w857 w858 w859 w860] -> w849
              frame 1, Default {
                n534 = local read "浓度1"() -> (w856:dbl)
              }
              frame 2 {
                n535 = local read "浓度2"() -> (w857:dbl)
              }
              frame 3 {
                n536 = local read "浓度3"() -> (w858:dbl)
              }
              frame 4 {
                n537 = local read "浓度4"() -> (w859:dbl)
              }
              frame 5 {
                n538 = local read "浓度5"() -> (w860:dbl)
              }
            }
            n539 = Not Equal To 0?(x=w849) -> (x != 0?=w848:bool)
            n540 = case shown="假" w848 {
              tunnel: [u16 8 ("address") u16 9 ("address")] -> w853
              tunnel: ["校零" ("测量模式") "校标" ("测量模式")] -> w843
              frame False {
              }
              frame True {
              }
            }
            n541 = global write "COD测量模式全局.vi" "测量模式"(w843) -> ()
            n542 = Insert Into Array(array=u16[] [] ("values"), index=0 ("索引"), new element=w853) -> (w847:u16[])
            n543 = Bundle By Name(cluster=cluster{"starting address":u16, "values":u16[]} {"starting address"=0, "values"=[]}, "starting address"=u16 4608 ("address"), "values"=w847) -> (w855:cluster{"starting address":u16, "values":u16[]})
            n544 = Enqueue Element(queue=w845, element=w855, error in (no error)=w844) -> ()  [unwired: 1 in, 3 out]
          }
          frame #2 {
            n545 = local write "枚举"(enum16{"读取数据", "写入数据", "读取写入DATABASE", "读取参数"}."写入数据" ("枚举")) -> ()
            n546 = call <vilib>:"Application Directory.vi"() -> ("Application Directory"=w872:path)
            n547 = Build Path(base path=w872, name or relative path="data\\Set.ini" ("名称或相对路径")) -> (appended path=w874:path)
            n548 = local read "当前校准"() -> (w867:i32)
            n549 = call <vilib>:"Open Config Data.vi"("configuration file path"=w874) -> ("error out"=w870:errorcluster, "refnum"=w871:T10)  [unwired: 8 in, 1 out]
            n550 = call-poly <vilib>:"Write Key.vi"("section"="CODMn", "error in (no error)"=w870, "value"=w867, "key"="当前选用的校准" ("section"), "refnum"=w871) -> ("error out"=w865:errorcluster, "refnum out"=w866:T10)  [unwired: 4 in, 1 out]
            n551 = call <vilib>:"Close Config Data.vi"("error in (no error)"=w865, "refnum"=w866) -> ()  [unwired: 8 in, 2 out]
          }
        }
      }
      event "自动切换量程", "低切高阈值", "高切低阈值": Value Change {
        w880 = "CODMn是否切换量程" ("key")
        n552 = event-data() -> ()  [unwired: 1 in, 6 out]
        n553 = call <vilib>:"Application Directory.vi"() -> ("Application Directory"=w893:path)
        n554 = Build Path(base path=w893, name or relative path="data\\Set.ini" ("名称或相对路径")) -> (appended path=w891:path)
        n555 = local read "自动切换量程"() -> (w887:enum16{"关闭", "自动切换测一次", "自动切换测两次"})
        n556 = call <vilib>:"Open Config Data.vi"("configuration file path"=w891) -> ("error out"=w889:errorcluster, "refnum"=w890:T10)  [unwired: 8 in, 1 out]
        n557 = call-poly <vilib>:"Write Key.vi"("section"=w880, "error in (no error)"=w889, "value"=w887, "key"="自动切换量程", "refnum"=w890) -> ("error out"=w883:errorcluster, "refnum out"=w884:T10)  [unwired: 4 in, 1 out]
        n558 = local read "低切高阈值"() -> (w879:dbl)
        n559 = call-poly <vilib>:"Write Key.vi"("section"=w880, "error in (no error)"=w883, "value"=w879, "key"="低切高阈值", "refnum"=w884) -> ("error out"=w881:errorcluster, "refnum out"=w882:T10)  [unwired: 4 in, 1 out]
        n560 = local read "高切低阈值"() -> (w878:dbl)
        n561 = call-poly <vilib>:"Write Key.vi"("section"=w880, "error in (no error)"=w881, "value"=w878, "key"="高切低阈值", "refnum"=w882) -> ("error out"=w876:errorcluster, "refnum out"=w877:T10)  [unwired: 4 in, 1 out]
        n562 = call <vilib>:"Close Config Data.vi"("error in (no error)"=w876, "refnum"=w877) -> ()  [unwired: 8 in, 2 out]
      }
      event "模型": Value Change {
        n563 = event-data() -> ()  [unwired: 1 in, 6 out]
        n564 = call <vilib>:"Application Directory.vi"() -> ("Application Directory"=w903:path)
        n565 = Build Path(base path=w903, name or relative path="data\\Set.ini" ("名称或相对路径")) -> (appended path=w901:path)
        n566 = call <vilib>:"Open Config Data.vi"("configuration file path"=w901) -> ("error out"=w899:errorcluster, "refnum"=w900:T10)  [unwired: 8 in, 1 out]
        n567 = local read "模型"() -> (w894:enum32{"线性", "多项式"})
        n568 = call-poly <vilib>:"Write Key.vi"("section"="CODMn模型选择" ("key"), "error in (no error)"=w899, "value"=w894, "key"="线性和多项式", "refnum"=w900) -> ("error out"=w895:errorcluster, "refnum out"=w896:T10)  [unwired: 4 in, 1 out]
        n569 = call <vilib>:"Close Config Data.vi"("error in (no error)"=w895, "refnum"=w896) -> ()  [unwired: 8 in, 2 out]
      }
      event "浓度1", "浓度2", "浓度3", "泵滴定数1", "泵滴定数2", "泵滴定数3", "启用1", "启用2", "启用3", "浓度4", "浓度5", "泵滴定数4", "泵滴定数5", "启用4", "启用5": Value Change {
        n570 = event-data() -> ()  [unwired: 1 in, 6 out]
        n571 = local read "选用水样"() -> (w919:enum16{"葡萄糖", "草酸钠"})
        n572 = local read "量程选择"() -> (w918:enum16{"低量程", "高量程", "0-2量程"})
        n573 = case shown="\"0-2量程\"" w918 {
          tunnel: ["低量程" "高量程" "0-2量程"] -> w916
          frame "低量程", Default {
          }
          frame "高量程" {
          }
          frame "0-2量程" {
          }
        }
        n574 = call <vilib>:"Application Directory.vi"() -> ("Application Directory"=w978:path)
        n575 = case shown="\"葡萄糖\", 默认" w919 {
          tunnel: ["葡萄糖标线" ("section") "草酸钠标线" ("section")] -> w925
          frame "葡萄糖", Default {
          }
          frame "草酸钠" {
          }
        }
        n576 = Build Path(base path=w978, name or relative path="data\\Set.ini" ("名称或相对路径")) -> (appended path=w976:path)
        n577 = call <vilib>:"Open Config Data.vi"("configuration file path"=w976) -> ("error out"=w974:errorcluster, "refnum"=w975:T10)  [unwired: 8 in, 1 out]
        n578 = local read "浓度1"() -> (w972:dbl)
        n579 = Concatenate Strings(w925, w916) -> (w917:string)
        n580 = local read "浓度2"() -> (w956:dbl)
        n581 = call-poly <vilib>:"Write Key.vi"("section"=w917, "error in (no error)"=w974, "value"=w972, "key"="浓度1", "refnum"=w975) -> ("error out"=w971:errorcluster, "refnum out"=w970:T10)  [unwired: 4 in, 1 out]
        n582 = local read "浓度3"() -> (w952:dbl)
        n583 = call-poly <vilib>:"Write Key.vi"("section"=w917, "error in (no error)"=w971, "value"=w956, "key"="浓度2", "refnum"=w970) -> ("error out"=w969:errorcluster, "refnum out"=w968:T10)  [unwired: 4 in, 1 out]
        n584 = local read "泵滴定数1"() -> (w950:dbl)
        n585 = call-poly <vilib>:"Write Key.vi"("section"=w917, "error in (no error)"=w969, "value"=w952, "key"="浓度3", "refnum"=w968) -> ("error out"=w967:errorcluster, "refnum out"=w966:T10)  [unwired: 4 in, 1 out]
        n586 = call-poly <vilib>:"Write Key.vi"("section"=w917, "error in (no error)"=w967, "value"=w950, "key"="泵滴定数1", "refnum"=w966) -> ("error out"=w965:errorcluster, "refnum out"=w964:T10)  [unwired: 4 in, 1 out]
        n587 = local read "泵滴定数2"() -> (w948:dbl)
        n588 = call-poly <vilib>:"Write Key.vi"("section"=w917, "error in (no error)"=w965, "value"=w948, "key"="泵滴定数2", "refnum"=w964) -> ("error out"=w963:errorcluster, "refnum out"=w962:T10)  [unwired: 4 in, 1 out]
        n589 = local read "泵滴定数3"() -> (w946:dbl)
        n590 = local read "浓度4"() -> (w915:dbl)
        n591 = call-poly <vilib>:"Write Key.vi"("section"=w917, "error in (no error)"=w963, "value"=w946, "key"="泵滴定数3", "refnum"=w962) -> ("error out"=w961:errorcluster, "refnum out"=w960:T10)  [unwired: 4 in, 1 out]
        n592 = local read "浓度5"() -> (w914:dbl)
        n593 = call-poly <vilib>:"Write Key.vi"("section"=w917, "error in (no error)"=w961, "value"=w915, "key"="浓度4", "refnum"=w960) -> ("error out"=w954:errorcluster, "refnum out"=w955:T10)  [unwired: 4 in, 1 out]
        n594 = call-poly <vilib>:"Write Key.vi"("section"=w917, "error in (no error)"=w954, "value"=w914, "key"="浓度5", "refnum"=w955) -> ("error out"=w912:errorcluster, "refnum out"=w913:T10)  [unwired: 4 in, 1 out]
        n595 = local read "泵滴定数4"() -> (w911:dbl)
        n596 = call-poly <vilib>:"Write Key.vi"("section"=w917, "error in (no error)"=w912, "value"=w911, "key"="泵滴定数4", "refnum"=w913) -> ("error out"=w959:errorcluster, "refnum out"=w958:T10)  [unwired: 4 in, 1 out]
        n597 = local read "泵滴定数5"() -> (w910:dbl)
        n598 = call-poly <vilib>:"Write Key.vi"("section"=w917, "error in (no error)"=w959, "value"=w910, "key"="泵滴定数5", "refnum"=w958) -> ("error out"=w908:errorcluster, "refnum out"=w909:T10)  [unwired: 4 in, 1 out]
        n599 = local read "启用1"() -> (w934:bool)
        n600 = call-poly <vilib>:"Write Key.vi"("section"=w917, "error in (no error)"=w908, "value"=w934, "key"="启用1", "refnum"=w909) -> ("error out"=w930:errorcluster, "refnum out"=w933:T10)  [unwired: 4 in, 1 out]
        n601 = local read "启用2"() -> (w931:bool)
        n602 = call-poly <vilib>:"Write Key.vi"("section"=w917, "error in (no error)"=w930, "value"=w931, "key"="启用2", "refnum"=w933) -> ("error out"=w941:errorcluster, "refnum out"=w940:T10)  [unwired: 4 in, 1 out]
        n603 = local read "启用3"() -> (w929:bool)
        n604 = call-poly <vilib>:"Write Key.vi"("section"=w917, "error in (no error)"=w941, "value"=w929, "key"="启用3", "refnum"=w940) -> ("error out"=w939:errorcluster, "refnum out"=w938:T10)  [unwired: 4 in, 1 out]
        n605 = local read "启用4"() -> (w904:bool)
        n606 = call-poly <vilib>:"Write Key.vi"("section"=w917, "error in (no error)"=w939, "value"=w904, "key"="启用4", "refnum"=w938) -> ("error out"=w937:errorcluster, "refnum out"=w936:T10)  [unwired: 4 in, 1 out]
        n607 = local read "启用5"() -> (w905:bool)
        n608 = call-poly <vilib>:"Write Key.vi"("section"=w917, "error in (no error)"=w937, "value"=w905, "key"="启用5", "refnum"=w936) -> ("error out"=w906:errorcluster, "refnum out"=w907:T10)  [unwired: 4 in, 1 out]
        n609 = local read "选用水样"() -> (w924:enum16{"葡萄糖", "草酸钠"})
        n610 = call-poly <vilib>:"Write Key.vi"("section"="标线选择", "error in (no error)"=w906, "value"=w924, "key"="选用水样", "refnum"=w907) -> ("error out"=w921:errorcluster, "refnum out"=w922:T10)  [unwired: 4 in, 1 out]
        n611 = call <vilib>:"Close Config Data.vi"("error in (no error)"=w921, "refnum"=w922) -> ()  [unwired: 8 in, 2 out]
      }
      event "读取": Value Change {
        n612 = event-data() -> ()  [unwired: 1 in, 6 out]
        n613 = local write "枚举"(enum16{"读取数据", "写入数据", "读取写入DATABASE", "读取参数"}."读取参数" ("枚举")) -> ()
        n614 = Bundle By Name(cluster=T5 {"starting address"=0, "number of holding registers"=0}, "starting address"=u16 4616, "number of holding registers"=u16 28) -> (w993:T5)
        n615 = Flush Queue(queue=w986, error in (no error)=w985) -> (queue out=w989:refnum<queue>, error out=w988:errorcluster)  [unwired: 1 out]
        n616 = Enqueue Element(queue=w989, element=w993, error in (no error)=w988) -> ()  [unwired: 1 in, 3 out]
        "读取KB值" <- TRUE
      }
      event "写入": Mouse Down {
        n617 = event-data() -> ()  [unwired: 1 in, 8 out]
        n618 = flat-sequence {
          tunnel: w994 -> [w997]
          frame #0 {
            n619 = local read "模型"() -> (w995:enum32{"线性", "多项式"})
            n620 = case shown="\"线性\", 默认" w995 {
              tunnel: [w1009 w1016] -> w999
              tunnel: w997 -> [w1003 w1015]
              tunnel: [w1003 w1015] -> w996
              frame "线性", Default {
                n621 = local read "K"() -> (w1006:dbl)
                n622 = local read "b"() -> (w1005:dbl)
                n623 = Build Array(w1006, w1005, 0.0 ("元素")) -> (w1004:dbl[])
                n624 = local read "量程选择"() -> (w1002:enum16{"低量程", "高量程", "0-2量程"})
                n625 = call "浮点转CDAB整形cod.vi"("浮点数"=w1004) -> ("CDAB整形输出"=w1007:u16[])  [unwired: 10 in]
                n626 = case shown="\"0-2量程\"" w1002 {
                  tunnel: [u16 4626 ("starting address") u16 4632 ("starting address") u16 4638 ("starting address")] -> w1001
                  frame "低量程", Default {
                  }
                  frame "高量程" {
                  }
                  frame "0-2量程" {
                  }
                }
                n627 = Bundle By Name(cluster=cluster{"starting address":u16, "values":u16[]} {"starting address"=4272, "values"=[]}, "starting address"=w1001, "values"=w1007) -> (w1009:cluster{"starting address":u16, "values":u16[]})
              }
              frame "多项式" {
                # "b,k,c"
                n628 = local read "多项式系数1"() -> (w1023:dbl[])
                n629 = local read "量程选择"() -> (w1013:enum16{"低量程", "高量程", "0-2量程"})
                n630 = Index Array(array=w1023) -> (element #1=w1018:dbl, element #2=w1019:dbl, element #3=w1014:dbl)  [unwired: 3 in]
                n631 = Build Array(w1019, w1018, w1014) -> (w1022:dbl[])
                n632 = case shown="\"0-2量程\"" w1013 {
                  tunnel: [u16 4626 ("starting address") u16 4632 ("starting address") u16 4638 ("starting address")] -> w1020
                  frame "低量程", Default {
                  }
                  frame "高量程" {
                  }
                  frame "0-2量程" {
                  }
                }
                n633 = call "浮点转CDAB整形cod.vi"("浮点数"=w1022) -> ("CDAB整形输出"=w1021:u16[])  [unwired: 10 in]
                n634 = Bundle By Name(cluster=cluster{"starting address":u16, "values":u16[]} {"starting address"=4272, "values"=[]}, "starting address"=w1020, "values"=w1021) -> (w1016:cluster{"starting address":u16, "values":u16[]})
              }
            }
            n635 = Enqueue Element(queue=w996, element=w999, timeout in ms (-1)=1000 ("超时毫秒(-1)")) -> ()  [unwired: 1 in, 3 out]
          }
          frame #1 {
            n636 = local write "枚举"(enum16{"读取数据", "写入数据", "读取写入DATABASE", "读取参数"}."写入数据" ("枚举")) -> ()
          }
        }
      }
      event "滴定曲线": Value Change {
        n637 = event-data() -> ()  [unwired: 1 in, 6 out]
        n638 = property on="窗格" class="Pane"("Origin"=T9 {"Horizontal"=0, "Vertical"=3200} ("原点")) -> ()  [unwired: 2 in, 2 out]
      }
      event "历史波形": Value Change {
        n639 = event-data() -> ()  [unwired: 1 in, 6 out]
        n640 = call-poly <vilib>:"Read Waveforms from File.vi"() -> ("error out"=w1029:errorcluster, "first waveform in record"=w1030:waveform(dbl))  [unwired: 6 in, 2 out]
        n641 = case shown="无错误" w1029 {
          tunnel: w1030 -> [w1033 _]
          frame No Error {
            n642 = Unbundle By Name(w1033) -> ("t0"=→"波形时间":timestamp, "Y"=w1032:dbl[])  [unwired: 2 out]
            n643 = local write "ORP滴定曲线2"(w1032) -> ()
            n644 = local write "滴定数-ORP值"(w1032) -> ()
          }
          frame Error {
            n645 = One Button Dialog(message="打开失败" ("消息")) -> ()  [unwired: 1 in, 1 out]
          }
        }
      }
    }
  }
  n646 = while {
    tunnel: w32 -> [w1172]
    tunnel: w31 -> [w1171]
    tunnel: w22 -> [w1167]
    tunnel: w21 -> [w1166]
    stop <- FALSE stop-if-true
    w1099 = T14 0 items=["最小二乘", "最小绝对残差", "Bisquare"] ("method")
    n647 = local read "自动切换量程"() -> (w1044:enum16{"关闭", "自动切换测一次", "自动切换测两次"})
    n648 = local read "浓度5"() -> (w1069:dbl)
    n649 = local read "浓度4"() -> (w1070:dbl)
    n650 = local read "浓度2"() -> (w1110:dbl)
    n651 = local read "浓度3"() -> (w1111:dbl)
    n652 = local read "浓度1"() -> (w1109:dbl)
    n653 = local read "泵滴定数3"() -> (w1114:dbl)
    n654 = Wait (ms)(milliseconds to wait=u32 500 ("等待时间（毫秒）")) -> ()  [unwired: 1 out]
    n655 = local read "泵滴定数2"() -> (w1113:dbl)
    n656 = local read "泵滴定数4"() -> (w1068:dbl)
    n657 = local read "泵滴定数5"() -> (w1067:dbl)
    n658 = local read "泵滴定数1"() -> (w1112:dbl)
    n659 = Not Equal To 0?(x=w1044) -> (x != 0?=w1043:bool)
    n660 = global read "CODMn断电保存全局变量.vi" "CODMn空白测试选择"() -> (w1046:enum16{"空白测试走纯水管", "空白测试走标样管"})
    n661 = Bundle By Name(cluster=T5 {"starting address"=4224, "number of holding registers"=16}, "starting address"=u16 4224, "number of holding registers"=u16 50) -> (w1225:T5)
    n662 = local read "基本量程"() -> (w1082:enum16{"10mg/L", "20mg/L"})
    n663 = Build Array("启用1", "启用2", "启用3", "启用4", "启用5") -> (w1058:bool[])
    n664 = Build Array(w1109, w1110, w1111, w1070, w1069) -> (w1101:dbl[])
    n665 = Build Array(w1112, w1113, w1114, w1068, w1067) -> (w1100:dbl[])
    n666 = Multiply(x="浓度 2", y=100.0) -> (x*y=w1147:dbl)
    n667 = Multiply(x="修正系数 2", y=100.0) -> (x*y=w1144:dbl)
    n668 = Select(t=T11."Enabled" ("禁用"), s=w1043, f=T11."Disabled and Grayed Out" ("禁用")) -> (s? t:f=w1064:T11)
    n669 = Multiply(x="温度", y=10.0) -> (x*y=w1150:dbl)
    n670 = global write "COD浓度全局变量.vi" "跨度液浓度"("跨度液浓度") -> ()
    n671 = call "线性公式CODMn用.vi"("标液浓度"=w1101, "监测浓度"=w1100, "启用"=w1058, "method"=w1099, "模型"="模型", "精度"=6) -> ("拟合方程"=→"拟合公式":string, "r^2"=→"r^2":dbl, "slope"=→"K":dbl, "intercept"=→"b":dbl, "XY图"=→"XY图":cluster{"X Values":dbl[], "Y Values":dbl[]}[], "Polynomial Coefficients"=→"多项式系数1":dbl[])  [unwired: 8 in]
    n672 = global write "COD浓度全局变量.vi" "基本量程"(w1082) -> ()
    n673 = local write "CODMn空白测试选择"(w1046) -> ()
    n674 = local write "修正系数"(w1144) -> ()
    n675 = local write "温度 2"(w1150) -> ()
    n676 = property on="低切高阈值" class="DigNum (严格)"("DisabledEnum"=w1064) -> ()  [unwired: 2 in, 2 out]
    n677 = property on="高切低阈值" class="DigNum (严格)"("DisabledEnum"=w1064) -> ()  [unwired: 2 in, 2 out]
    n678 = local write "浓度"(w1147) -> ()
    n679 = Enqueue Element(queue=w1172, element=w1225, error in (no error)=w1171) -> ()  [unwired: 1 in, 3 out]
    n680 = local read "Registers"() -> (w1091:u16[])
    n681 = To Word Integer(number=w1091) -> (16bit integer=w1090:i16[])
    n682 = Index Array(array=w1090, index #1=0 ("索引"), index #4=3 ("索引"), index #14=13 ("索引"), index #15=14 ("索引"), index #21=20 ("索引"), index #32=31 ("索引")) -> (element #1=w1141:i16, element #2=w1140:i16, element #3=w1139:i16, element #4=w1057:i16, element #5=→"模式（受控）":i16, element #6=→"进样管":i16, element #7=→"高锰酸钾":i16, element #8=→"草酸钠":i16, element #9=→"硫酸":i16, element #10=w1089:i16, element #11=w1199:i16, element #12=w1054:i16, element #13=w1081:i16, element #14=w1216:i16, element #15=w1174:i16, element #16=w1040:i16, element #21=w1036:i16, element #33=→"分":i16, element #34=→"秒":i16)  [unwired: 28 in, 15 out]
    "多列列表框" <- w1040
    n683 = local write "基本量程"(w1036) -> ()
    n684 = Number To Decimal String(number=w1036) -> (decimal integer string=→"基本量程(显示)":string)  [unwired: 1 in]
    n685 = Build Array(w1141, w1140, w1139) -> (w1142:i16[])
    n686 = To Single Precision Float(number=w1089) -> (single precision float=→"ORP显示":sgl)
    n687 = Divide(x=w1174, y=u16 1000) -> (x/y=→"标度滴定值":dbl)
    n688 = Divide(x=w1199, y=u16 10) -> (x/y=→"温度":dbl)
    n689 = Equal?(x=w1054, y=u16 2) -> (x = y?=→"断电排液标记":bool)
    n690 = global write "COD测量模式全局.vi" "CODMn工作状态"(w1057) -> ()
    n691 = Equal?(x=w1081, y=u16 2) -> (x = y?=w1079:bool)
    "温控器故障" <- w1079
    n692 = Equal?(x=w1081, y=u16 3) -> (x = y?=w1078:bool)
    "加热故障" <- w1078
    n693 = Equal?(x=w1081, y=u16 4) -> (x = y?=w1077:bool)
    "高锰酸钾报警" <- w1077
    n694 = Equal?(x=w1081, y=u16 5) -> (x = y?=w1076:bool)
    "草酸钠报警" <- w1076
    n695 = Equal?(x=w1081, y=u16 6) -> (x = y?=w1075:bool)
    "测量错误" <- w1075
    n696 = Equal?(x=w1081, y=u16 8) -> (x = y?=w1074:bool)
    "校零错误" <- w1074
    n697 = Equal?(x=w1081, y=u16 7) -> (x = y?=w1073:bool)
    "校标错误" <- w1073
    n698 = Equal?(x=w1081, y=u16 9) -> (x = y?=w1072:bool)
    "进水样超量程" <- w1072
    n699 = Divide(x=w1216, y=u16 1000) -> (x/y=→"零点滴定值":dbl)
    n700 = Equal?(x=w1081, y=u16 10) -> (x = y?=w1071:bool)
    "排液故障" <- w1071
    n701 = Equal?(x=w1054, y=u16 1) -> (x = y?=→"排液标记":bool)
    n702 = global write "运行时序全局变量.vi" "多列列表框"(w1040) -> ()
    n703 = Equal?(x=w1081, y=u16 1) -> (x = y?=w1080:bool)
    "ORP故障" <- w1080
    n704 = Equal?(x=w1057, y=u16 0) -> (x = y?=→"待机":bool)
    n705 = Equal?(x=w1057, y=u16 8) -> (x = y?=→"校零标记":bool)
    n706 = Equal?(x=w1057, y=u16 9) -> (x = y?=→"校标标记":bool)
    n707 = Equal?(x=w1057, y=u16 1) -> (x = y?=→"水样测量":bool)
    n708 = Equal?(x=w1057, y=u16 7) -> (x = y?=→"质控样测量":bool)
    n709 = Equal?(x=w1057, y=u16 10) -> (x = y?=→"加标回收测量":bool)
    n710 = Equal?(x=w1057, y=u16 2) -> (x = y?=→"标样核查标记":bool)
    n711 = Equal?(x=w1057, y=u16 6) -> (x = y?=→"平行样测量":bool)
    n712 = Equal?(x=w1057, y=u16 3) -> (x = y?=→"零点核查标记":bool)
    n713 = Equal?(x=w1057, y=u16 4) -> (x = y?=→"跨度核查标记":bool)
    n714 = Equal?(x=w1057, y=u16 5) -> (x = y?=→"空白测试标记":bool)
    n715 = feedback #2(w1040) -> (w1157:i16)
    n716 = feedback-in #2(w1040) -> ()
    n717 = Compound Arithmetic op=OR ("复合运算")(w1080, w1079, w1078, w1077, w1076, w1075, w1073, w1074, w1072, w1071) -> (→"故障标记":bool)
    n718 = Not Equal?(x=w1040, y=w1157) -> (x != y?=w1156:bool)
    n719 = Bundle By Name(cluster=T3 {"ORP故障"=FALSE, "温控器故障"=FALSE, "加热故障"=FALSE, "高锰酸钾报警"=FALSE, "草酸钠报警"=FALSE, "测量错误"=FALSE, "校零错误"=FALSE, "校标错误"=FALSE, " 进水样超量程"=FALSE, "排液阀故障"=FALSE} ("报警簇"), "ORP故障"=w1080, "温控器故障"=w1079, "加热故障"=w1078, "高锰酸钾报警"=w1077, "草酸钠报警"=w1076, "测量错误"=w1075, "校零错误"=w1074, "校标错误"=w1073, "进水样超量程"=w1072, "排液阀故障"=w1071) -> (w1158:T3)
    "报警簇" <- w1158
    n720 = local read "断电排液标记"() -> (w1052:bool)
    n721 = call "HexToDate.vi"("数组"=w1142) -> ("DATE"=w1137:timestamp[])  [unwired: 10 in]
    n722 = Index Array(array=w1137) -> (element=→"仪器时间":timestamp)  [unwired: 1 in]
    n723 = First Call?() -> (First Call?: T/F=w1050:bool)
    n724 = Get Date/Time In Seconds() -> (seconds since 1Jan1904=w1136:timestamp)
    "系统时间" <- w1136
    n725 = call <vilib>:"Boolean Crossing PtByPt.vi"("direction"=enum16{"either", "false-true", "true-false"}."false-true", "input"=w1052) -> ("crossing"=w1051:bool)  [unwired: 1 in]
    n726 = call "CODMn报警信息.vi"("报警簇"=w1158) -> ("CODMN报警信息"=w1159:string)  [unwired: 10 in]
    n727 = case shown="假" w1050 {
      tunnel: w1156 -> [w1230 _]
      tunnel: w1040 -> [w1229 _]
      frame False {
        n728 = case shown="真" w1230 {
          tunnel: w1229 -> [_ w1242]
          frame False {
          }
          frame True {
            n729 = property on="多列列表框" class="MCListbox (严格)"() -> ("ItemNames"=w1236:string[][])  [unwired: 2 in, 2 out]
            n730 = Index Array(array=w1236, index (row)=w1242) -> (element=w1233:string[])  [unwired: 1 in]
            n731 = Index Array(array=w1233, index=0 ("索引")) -> (element=w1231:string)
            n732 = Array To Spreadsheet String(delimiter (Tab)="-" ("分隔符(Tab)"), array=w1233, 3:"" ("格式字符串")) -> ()  [unwired: 1 out]
            n733 = Get Date/Time In Seconds() -> (seconds since 1Jan1904=w1240:timestamp)
            n734 = Bundle(cluster=T12 {"时间标识"=timestamp(0 s since 1904-01-01), "参数"="", "日志信息"="", "流程参数"=""} ("data in"), "时间标识"=w1240, "参数"="CODMn" ("table输入"), "日志信息"=w1231, "流程参数"="" ("table输入")) -> (w1237:T12)
            n735 = call "流程日志字段定义.vi"("table输入"="操作日志", "data in"=w1237) -> ("table输出"=w1245:string, "columns"=w1246:string[], "data out"=w1247:T15)  [unwired: 7 in]
            n736 = call "插入数据.vi"("data"=w1247, "columns"=w1246, "database"="database3.mdb", "table"=w1245) -> ()  [unwired: 7 in, 1 out]
          }
        }
      }
      frame True {
      }
    }
    n737 = case shown="真" w1051 {
      frame False {
      }
      frame True {
        n738 = Get Date/Time In Seconds() -> (seconds since 1Jan1904=w1253:timestamp)
        n739 = Bundle(cluster=T12 {"时间标识"=timestamp(0 s since 1904-01-01), "参数"="", "日志信息"="", "流程参数"=""} ("data in"), "时间标识"=w1253, "参数"="CODMn" ("table输入"), "日志信息"="断电排液", "流程参数"="" ("table输入")) -> (w1251:T12)
        n740 = call "流程日志字段定义.vi"("table输入"="操作日志", "data in"=w1251) -> ("table输出"=w1256:string, "columns"=w1257:string[], "data out"=w1258:T15)  [unwired: 7 in]
        n741 = call "插入数据.vi"("data"=w1258, "columns"=w1257, "database"="database3.mdb", "table"=w1256) -> ()  [unwired: 7 in, 1 out]
      }
    }
    n742 = Greater?(x=w1040, y=u16 0) -> (0:w1039:bool)
    n743 = Less Or Equal?(x=w1040, y=u16 4) -> (x <= y?=w1107:bool)
    n744 = Equal?(x=w1040, y=u16 5) -> (x = y?=w1170:bool)
    n745 = feedback #3(w1159) -> (w1160:string)
    n746 = feedback-in #3(w1159) -> ()
    n747 = Greater?(x=w1040, y=u16 0) -> (0:w1104:bool)
    n748 = Not Equal?(x=w1159, y="") -> (x != y?=w1164:bool)
    n749 = And(x=w1039, y=w1107) -> (x .and. y?=w1042:bool)
    n750 = global read "COD读取DATA全局.vi" "data"() -> (w1120:T16)
    n751 = call <vilib>:"Boolean Crossing PtByPt.vi"("direction"=enum16{"either", "false-true", "true-false"}."false-true", "input"=w1170) -> ("crossing"=w1168:bool)  [unwired: 1 in]
    n752 = call <vilib>:"Boolean Crossing PtByPt.vi"("direction"=enum16{"either", "false-true", "true-false"}."false-true", "input"=w1104) -> ("crossing"=w1103:bool)  [unwired: 1 in]
    n753 = Build Array(w1136) -> (w1135:timestamp[])
    n754 = Not Equal?(x=w1159, y=w1160) -> (x != y?=w1161:bool)
    n755 = case shown="真" w1168 {
      tunnel: w1167 -> [_ w1339]
      tunnel: w1166 -> [_ w1334]
      frame False {
      }
      frame True {
        n756 = Bundle By Name(cluster=T5 {"starting address"=0, "number of holding registers"=0}, "starting address"=u16 4101, "number of holding registers"=u16 10) -> (w1338:T5)
        n757 = Enqueue Element(queue=w1339, element=w1338, error in (no error)=w1334) -> ()  [unwired: 1 in, 3 out]
        n758 = local write "枚举"(enum16{"读取数据", "写入数据", "读取写入DATABASE", "读取参数"}."读取写入DATABASE" ("枚举")) -> ()
      }
    }
    n759 = case shown="真" w1042 {
      frame False {
      }
      frame True {
        n760 = local read "测量模式数字"() -> (w1268:i32)
        n761 = local read "标样核查标记"() -> (w1271:bool)
        n762 = local read "零点核查标记"() -> (w1270:bool)
        n763 = local read "跨度核查标记"() -> (w1266:bool)
        n764 = local read "空白测试标记"() -> (w1265:bool)
        n765 = local read "加标回收测量"() -> (w1264:bool)
        n766 = local read "平行样测量"() -> (w1263:bool)
        n767 = local read "启动时间"() -> (w1260:timestamp)
        n768 = local read "水样测量"() -> (w1272:bool)
        n769 = local read "校零标记"() -> (w1262:bool)
        n770 = local read "校标标记"() -> (w1261:bool)
        n771 = case shown="0, 默认" w1268 {
          tunnel: ["水样测试" ("测量模式") "标样核查" ("测量模式") "零点核查" ("测量模式") "跨度核查" ("测量模式") "空白测试" ("测量模式") "加标回收" ("测量模式") "平行样" ("测量模式") "校零" ("测量模式") "校标" ("测量模式")] -> w1267
          tunnel: w1260 -> [w1273 _ _ _ _ w1279 _ _ _]
          frame 0, Default {
            n772 = global write "COD测量模式全局.vi" "水样启动时间"(w1273) -> ()
          }
          frame 1 {
          }
          frame 2 {
          }
          frame 3 {
          }
          frame 4 {
          }
          frame 5 {
            n773 = global write "COD测量模式全局.vi" "加标回收启动时间"(w1279) -> ()
          }
          frame 6 {
          }
          frame 7 {
          }
          frame 8 {
          }
        }
        n774 = Build Array(w1272, w1271, w1270, w1266, w1265, w1264, w1263, w1262, w1261) -> (w1269:bool[])
        n775 = for {
          tunnel: w1269 -> [w1285] mode=indexing
          i -> [w1284]
          n776 = case shown="真" w1285 {
            tunnel: w1284 -> [_ w1286]
            frame False {
            }
            frame True {
              "测量模式数字" <- w1286
            }
          }
        }
        n777 = global write "COD测量模式全局.vi" "测量模式"(w1267) -> ()
      }
    }
    n778 = case shown="真" w1103 {
      frame False {
      }
      frame True {
        n779 = Get Date/Time In Seconds() -> (seconds since 1Jan1904=→"启动时间":timestamp)
      }
    }
    n780 = global read "COD测量模式全局.vi" "测量模式"() -> (w1038:string)
    "测量模式(显示)" <- w1038
    n781 = call "DateToHex.vi"("DATE"=w1135) -> ("数组"=w1134:u16[])  [unwired: 10 in]
    n782 = call "DateToHex.vi"("DATE"=w1137) -> ("数组"=w1129:u16[])  [unwired: 10 in]
    n783 = And(x=w1161, y=w1164) -> (x .and. y?=w1162:bool)
    n784 = Unbundle By Name(w1120) -> ("时间"=w1119:timestamp, "检测值"=w1118:sgl, "数据标识"=w1117:string)
    n785 = case shown="真" w1162 {
      tunnel: w1159 -> [_ w1323]
      frame False {
      }
      frame True {
        n786 = Get Date/Time In Seconds() -> (seconds since 1Jan1904=w1325:timestamp)
        n787 = Bundle By Name(cluster=T13 {"时间标识"=timestamp(0 s since 1904-01-01), "设备"="", "日志信息"=""} ("data in"), "时间标识"=w1325, "设备"="CODMn", "日志信息"=w1323) -> (w1326:T13)
        n788 = call "报警信息字段定义.vi"("table输入"="报警信息", "data in"=w1326) -> ("table输出"=w1330:string, "columns"=w1331:string[], "data out"=w1332:T13)  [unwired: 7 in]
        n789 = call "插入数据.vi"("data"=w1332, "columns"=w1331, "database"="database3.mdb", "table"=w1330) -> ()  [unwired: 7 in, 1 out]
      }
    }
    n790 = Index Array(array=w1129, index=2 ("索引")) -> (element=w1131:u16)
    n791 = Index Array(array=w1134, index=2 ("索引")) -> (element=w1132:u16)
    n792 = local read "测量数据区"() -> (w1121:T2)
    n793 = case shown="\"水样测试\"" w1038 {
      tunnel: w1121 -> [w1287 w1292 w1297 w1302 w1307 w1312 w1317 w1322]
      tunnel: [w1287 w1291 w1293 w1301 w1306 w1311 w1313 w1321] -> w1045
      tunnel: w1119 -> [_ w1290 w1296 w1300 w1305 w1310 w1316 w1320]
      tunnel: w1118 -> [_ w1289 w1295 w1299 w1304 w1309 w1315 w1319]
      tunnel: w1117 -> [_ w1288 w1294 w1298 w1303 w1308 w1314 w1318]
      frame "", Default {
      }
      frame "水样测试" {
        n794 = Bundle By Name(cluster=w1292, "水样数据时间"=w1290, "水样实测值"=w1289, "水样数据标识"=w1288) -> (w1291:T2)
      }
      frame "标样核查" {
        n795 = Bundle By Name(cluster=w1297, "跨度核查数据时间"=w1296, "跨度核查实测值"=w1295, "跨度核查数据标识"=w1294) -> (w1293:T2)
      }
      frame "零点核查" {
        n796 = Bundle By Name(cluster=w1302, "零点核查数据时间"=w1300, "零点核查实测值"=w1299, "零点核查数据标识"=w1298) -> (w1301:T2)
      }
      frame "加标回收" {
        n797 = Bundle By Name(cluster=w1307, "加标回收数据时间"=w1305, "加标回收实测值"=w1304, "加标回收数据标识"=w1303) -> (w1306:T2)
      }
      frame "平行样" {
        n798 = Bundle By Name(cluster=w1312, "平行样数据时间"=w1310, "平行样实测值"=w1309, "平行样数据标识"=w1308) -> (w1311:T2)
      }
      frame "校零" {
        n799 = Bundle By Name(cluster=w1317, "空白数据时间"=w1316, "空白实测值"=w1315, "空白数据标识"=w1314) -> (w1313:T2)
      }
      frame "校标" {
        n800 = Bundle By Name(cluster=w1322, "标样数据时间"=w1320, "标样实测值"=w1319, "标样数据标识"=w1318) -> (w1321:T2)
      }
    }
    "测量数据区" <- w1045
    n801 = Split Number(x=w1131) -> (hi(x)=w1125:u8)  [unwired: 1 out]
    n802 = Split Number(x=w1132) -> (hi(x)=w1128:u8)  [unwired: 1 out]
    n803 = To Byte Integer(number=w1125) -> (8bit integer=w1124:i8)
    n804 = To Byte Integer(number=w1128) -> (8bit integer=w1127:i8)
    n805 = Subtract(x=w1124, y=w1127) -> (x-y=w1126:i8)
    n806 = local read "通讯状态"() -> (w1048:bool)
    n807 = Absolute Value(x=w1126) -> (abs(x)=w1123:i8)
    n808 = Greater Or Equal?(x=w1123, y=i8 1) -> (x >= y?=w1049:bool)
    n809 = global write "COD读取DATA全局.vi" "测量数据区"(w1045) -> ()
    n810 = And(x=w1049, y=w1048) -> (x .and. y?=w1047:bool)
    n811 = case shown="真" w1047 {
      frame False {
      }
      frame True {
        n812 = flat-sequence {
          frame #0 {
            n813 = property on="时间校准" class="Bool (严格)"("Val(Sgnl)"=TRUE ("值(信号)")) -> ()  [unwired: 2 in, 2 out]
          }
          frame #1 {
            n814 = Wait (ms)(milliseconds to wait=u32 500 ("等待时间（毫秒）")) -> ()  [unwired: 1 out]
          }
          frame #2 {
            n815 = property on="时间校准" class="Bool (严格)"("Val(Sgnl)"=FALSE ("值(信号)")) -> ()  [unwired: 2 in, 2 out]
          }
        }
      }
    }
  }
  n816 = while {
    tunnel: w2 -> [w1356]
    tunnel: w1 -> [w1355]
    tunnel: w18 -> [w1354]
    tunnel: w32 -> [w1353]
    tunnel: w31 -> [w1352]
    tunnel: [w1342] -> w30
    tunnel: [w1351] -> w29
    tunnel: w15 -> [w1349]
    tunnel: w14 -> [w1348]
    tunnel: w22 -> [w1347]
    tunnel: w21 -> [w1346]
    tunnel: w20 -> [w1345]
    tunnel: w18 -> [w1340]
    stop <- FALSE stop-if-true
    n817 = case shown="\"读取参数\"" "枚举" {
      tunnel: w1356 -> [w1392 w1403 w1487 w1699]
      tunnel: w1355 -> [w1391 w1399 w1486 w1698]
      tunnel: w1354 -> [_ w1402 _ _]
      tunnel: [w1359 w1401 w1489 w1693] -> w1351
      tunnel: [w1358 w1400 w1488 w1691] -> w1342
      tunnel: w1353 -> [w1389 _ _ _]
      tunnel: w1352 -> [w1385 _ _ _]
      tunnel: w1349 -> [_ _ _ w1697]
      tunnel: w1348 -> [_ _ _ w1696]
      tunnel: w1347 -> [_ _ w1485 _]
      tunnel: w1346 -> [_ _ w1484 _]
      tunnel: w1345 -> [_ w1398 _ _]
      tunnel: w1340 -> [_ _ w1454 _]
      frame "读取数据", Default {
        n818 = Dequeue Element(queue=w1389, timeout in ms (-1)=1000 ("超时毫秒(-1)"), error in (no error)=w1385) -> (element=w1388:T5)  [unwired: 3 out]
        n819 = Unbundle By Name(w1388) -> ("starting address"=w1387:u16, "number of holding registers"=w1386:u16)
        n820 = call <vilib>:"Read Holding Registers.vi"("error in (no error)"=w1391, "quantity"=w1386, "starting address"=w1387, "MB session in"=w1392) -> ("error out"=w1357:errorcluster, "Registers"=w1390:u16[], "MB session out"=w1383:refnum<class "MB_Master_Serial.lvclass">)  [unwired: 5 in]
        n821 = case shown="无错误" w1357 {
          tunnel: w1390 -> [w1393 _]
          frame No Error {
            "Registers" <- w1393
          }
          frame Error {
          }
        }
        n822 = call <vilib>:"Read Coils.vi"("error in (no error)"=w1357, "quantity"=u16 8, "starting address"=u16 140, "MB session in"=w1383) -> ("error out"=w1371:errorcluster, "Coils"=w1380:bool[], "MB session out"=w1372:refnum<class "MB_Master_Serial.lvclass">)  [unwired: 5 in]
        n823 = Index Array(array=w1380) -> (element #1=→"进水样":bool, element #2=→"进蒸馏水":bool, element #3=→"进标液":bool, element #4=→"进质控样":bool, element #5=→"进加标回收样":bool, element #6=→"进高锰酸钾":bool, element #7=→"进草酸钠":bool, element #8=→"进硫酸":bool)  [unwired: 9 in, 1 out]
        n824 = call <vilib>:"Read Coils.vi"("error in (no error)"=w1371, "quantity"=u16 1, "starting address"=u16 137, "MB session in"=w1372) -> ("error out"=w1367:errorcluster, "Coils"=w1361:bool[], "MB session out"=w1368:refnum<class "MB_Master_Serial.lvclass">)  [unwired: 5 in]
        n825 = Index Array(array=w1361) -> (element=→"搅拌":bool)  [unwired: 1 in]
        n826 = call <vilib>:"Read Coils.vi"("error in (no error)"=w1367, "quantity"=u16 1, "starting address"=u16 400, "MB session in"=w1368) -> ("error out"=w1358:errorcluster, "Coils"=w1364:bool[], "MB session out"=w1359:refnum<class "MB_Master_Serial.lvclass">)  [unwired: 5 in]
        n827 = Index Array(array=w1364) -> (element=→"加热":bool)  [unwired: 1 in]
      }
      frame "写入数据" {
        n828 = flat-sequence {
          tunnel: w1403 -> [w1414]
          tunnel: w1402 -> [w1413]
          tunnel: w1399 -> [w1407]
          tunnel: w1398 -> [w1406]
          tunnel: [w1409] -> w1397
          tunnel: [w1408] -> w1396
          tunnel: [w1405] -> w1395
          tunnel: [w1404] -> w1394
          tunnel: [w1415] -> w1400
          tunnel: [w1421] -> w1401
          tunnel: w1397 -> [w1421]
          tunnel: w1396 -> [w1415]
          tunnel: w1395 -> [w1420]
          tunnel: w1394 -> [w1419]
          frame #0 {
            n829 = Dequeue Element(queue=w1413, error in (no error)=w1406) -> (queue out=w1405:refnum<queue>, element=w1412:cluster{"starting address":u16, "values":u16[]}, error out=w1404:errorcluster)  [unwired: 1 in, 1 out]
            n830 = Unbundle By Name(w1412) -> ("starting address"=w1411:u16, "values"=w1410:u16[])
            n831 = call <vilib>:"Write Multiple Registers.vi"("error in (no error)"=w1407, "values"=w1410, "starting address"=w1411, "MB session in"=w1414) -> ("error out"=w1408:errorcluster, "MB session out"=w1409:refnum<class "MB_Master_Serial.lvclass">)  [unwired: 6 in]
          }
          frame #1 {
            n832 = Get Queue Status(queue=w1420, error in (no error)=w1419) -> (# elements in queue=w1418:i32)  [unwired: 1 in, 7 out]
            n833 = Equal To 0?(x=w1418) -> (x = 0?=w1417:bool)
            n834 = case shown="假" w1417 {
              tunnel: [enum16{"读取数据", "写入数据", "读取写入DATABASE", "读取参数"}."写入数据" ("枚举") enum16{"读取数据", "写入数据", "读取写入DATABASE", "读取参数"}."读取数据" ("枚举")] -> w1416
              tunnel: w1415 -> [_ w1423]
              frame False {
              }
              frame True {
                n835 = case shown="无错误" w1423 {
                  tunnel: ["保存成功" ("消息") "保存失败" ("消息")] -> _
                  frame No Error {
                  }
                  frame Error {
                  }
                }
              }
            }
            n836 = local write "枚举"(w1416) -> ()
          }
        }
      }
      frame "读取写入DATABASE" {
        n837 = Dequeue Element(queue=w1485, timeout in ms (-1)=1000 ("超时毫秒(-1)"), error in (no error)=w1484) -> (element=w1492:T5)  [unwired: 3 out]
        n838 = Unbundle By Name(w1492) -> ("starting address"=w1491:u16, "number of holding registers"=w1490:u16)
        n839 = call <vilib>:"Read Holding Registers.vi"("error in (no error)"=w1486, "quantity"=w1490, "starting address"=w1491, "MB session in"=w1487) -> ("error out"=w1488:errorcluster, "Registers"=w1443:u16[], "MB session out"=w1489:refnum<class "MB_Master_Serial.lvclass">)  [unwired: 5 in]
        n840 = To Word Integer(number=w1443) -> (16bit integer=w1442:i16[])
        n841 = Split 1D Array(array=w1442, index=3 ("索引")) -> (first subarray=w1482:i16[], second subarray=w1472:i16[])
        n842 = global read "CODMN外部API.vi" "CODMn外围API"() -> (w1428:T17)
        n843 = Unbundle By Name(w1428) -> ("运行模式"=w1427:enum16{"维护模式", "常规模式", "应急模式", "质控模式"})
        n844 = case shown="\"维护模式\", 默认" w1427 {
          tunnel: ["M" ("单位") "N" ("单位") "N" ("单位") "N" ("单位")] -> w1456
          frame "维护模式", Default {
          }
          frame "常规模式" {
          }
          frame "应急模式" {
          }
          frame "质控模式" {
          }
        }
        n845 = Index Array(array=w1482) -> (element #1=w1480:i16, element #2=w1479:i16, element #3=w1478:i16)  [unwired: 3 in]
        n846 = Index Array(array=w1472) -> (element #1=w1447:i16, element #2=w1476:i16, element #3=w1475:i16, element #4=w1474:i16, element #5=w1473:i16)  [unwired: 5 in]
        n847 = Index Array(array=w1472, index=6 ("索引")) -> (element=w1470:i16)
        n848 = To Single Precision Float(number=w1447) -> (single precision float=w1449:sgl)
        n849 = Divide(x=w1449, y=sgl 100.0) -> (x/y=w1448:sgl)
        n850 = Less Or Equal?(x=w1448, y=sgl 0.01) -> (x <= y?=w1451:bool)
        n851 = case shown="真" w1451 {
          tunnel: [w1682 w1683] -> w1450
          tunnel: w1448 -> [w1682 _]
          frame False {
          }
          frame True {
            n852 = Random Number (0-1)() -> (number: 0 to 1=w1686:dbl)
            n853 = Increment(x=w1686) -> (x+1=w1684:dbl)
            n854 = Divide(x=w1684, y=sgl 100.0) -> (x/y=w1683:dbl)
          }
        }
        n855 = Build Array(w1480, w1479, w1478) -> (w1477:i16[])
        n856 = To Single Precision Float(number=w1476) -> (single precision float=w1460:sgl)
        n857 = To Single Precision Float(number=w1470) -> (single precision float=w1453:sgl)
        n858 = To Single Precision Float(number=w1475) -> (single precision float=w1461:sgl)
        n859 = To Single Precision Float(number=w1474) -> (single precision float=w1462:sgl)
        n860 = To Single Precision Float(number=w1473) -> (single precision float=w1467:sgl)
        n861 = call "HexToDate.vi"("数组"=w1477) -> ("DATE"=w1481:timestamp[])  [unwired: 10 in]
        n862 = global read "COD测量模式全局.vi" "测量模式"() -> (w1437:string)
        n863 = Index Array(array=w1481) -> (element=w1438:timestamp)  [unwired: 1 in]
        n864 = Greater Than 0?(x="量程切换次数") -> (x > 0?=w1431:bool)
        n865 = case shown="\"标样核查\"" w1437 {
          selector: w1437 -> [w1639 _]
          tunnel: [w1639 w1641] -> w1436
          frame "", Default {
          }
          frame "标样核查" {
            n866 = global read "CODMn断电保存全局变量.vi" "CODMn空白测试选择"() -> (w1640:enum16{"空白测试走纯水管", "空白测试走标样管"})
            n867 = case shown="\"空白测试走标样管\"" w1640 {
              tunnel: ["标样核查" "空白测试"] -> w1641
              frame "空白测试走纯水管", Default {
              }
              frame "空白测试走标样管" {
              }
            }
          }
        }
        n868 = disable-structure shown="启用" {
          disable-tunnel: w1450 -> [w1645 w1669]
          disable-tunnel: [w1644 w1669] -> w1434
          frame Disabled {
            # "高量程0-5之间会乘1.2的系数\n低量程0-2之间会乘1.1的系数"
            n869 = property on="基本量程" class="Enum (严格)"() -> ("Value"=w1646:enum16{"10mg/L", "20mg/L"})  [unwired: 2 in, 2 out]
            n870 = case shown="\"10mg/L\", 默认" w1646 {
              tunnel: w1645 -> [w1649 w1659]
              tunnel: [w1647 w1658] -> w1644
              frame "10mg/L", Default {
                n871 = Less Or Equal?(x=w1649, y=2.0) -> (x <= y?=w1652:bool)
                n872 = Greater?(x=w1649, y=0.0) -> (0:w1651:bool)
                n873 = And(x=w1652, y=w1651) -> (x .and. y?=w1648:bool)
                n874 = case shown="真" w1648 {
                  tunnel: w1649 -> [w1654 w1657]
                  tunnel: [w1654 w1655] -> w1647
                  frame False {
                  }
                  frame True {
                    n875 = Multiply(x=w1657, y=1.1) -> (x*y=w1655:dbl)
                  }
                }
              }
              frame "20mg/L" {
                n876 = Greater?(x=w1659, y=0.0) -> (0:w1662:bool)
                n877 = Less Or Equal?(x=w1659, y=5.0) -> (x <= y?=w1663:bool)
                n878 = And(x=w1663, y=w1662) -> (x .and. y?=w1660:bool)
                n879 = case shown="真" w1660 {
                  tunnel: w1659 -> [w1665 w1668]
                  tunnel: [w1665 w1666] -> w1658
                  frame False {
                  }
                  frame True {
                    n880 = Multiply(x=w1668, y=1.2) -> (x*y=w1666:dbl)
                  }
                }
              }
            }
          }
          frame Enabled {
          }
        }
        "COD浓度（mg/L)" <- w1434
        n881 = local write "启动时间"(w1438) -> ()
        n882 = Format Date/Time String(seconds (now)=w1438) -> (date/time string=→"数据时间":string)  [unwired: 2 in]
        n883 = global read "COD测量模式全局.vi" "测量模式"() -> (w1441:string)
        n884 = case shown="\"跨度核查\"" w1441 {
          tunnel: [0.0 w1671 w1674] -> w1440
          frame "", Default {
          }
          frame "标样核查", "校标" {
            n885 = local read "标样浓度 2"() -> (w1672:dbl)
            n886 = Divide(x=w1672, y=100.0) -> (x/y=w1671:dbl)
          }
          frame "跨度核查" {
            n887 = local read "跨度液浓度"() -> (w1674:dbl)
          }
        }
        n888 = Divide(x=w1467, y=sgl 1000.0) -> (x/y=w1463:sgl)
        n889 = local read "故障标记"() -> (w1435:bool)
        n890 = local read "温度"() -> (w1455:dbl)
        n891 = local read "基本量程"() -> (w1429:enum16{"10mg/L", "20mg/L"})
        n892 = case shown="真" w1435 {
          tunnel: ["N" ("数据标识") "D" ("数据标识")] -> w1458
          frame False {
          }
          frame True {
          }
        }
        n893 = Format Into String(format string="w%05d" ("格式字符串"), u32 1019 ("因子编码")) -> (resulting string=w1459:string)  [unwired: 2 in, 1 out]
        n894 = Bundle(cluster=T16 {"时间"=timestamp(0 s since 1904-01-01), "测量模式"="", "数据类型"="", "检测值"=0.0, "单位"="", "数据标识"="", "因子编码"="", "标样参考值"=0.0, "ORP-A"=0.0, "ORP-B"=0.0, "ORP-K"=0.0, "COD滴定值"=0.0, "高锰酸钾滴定数"=0.0, "温度"=0.0, "量程"=0.0} ("data"), "时间"=w1438, "测量模式"=w1436, "数据类型"=w1456, "检测值"=w1434, "单位"="mg/L", "数据标识"=w1458, "因子编码"=w1459, "标样参考值"=w1440, "ORP-A"=w1460, "ORP-B"=w1461, "ORP-K"=w1462, "COD滴定值"=w1463, "高锰酸钾滴定数"=w1453, "温度"=w1455, "量程"=w1429) -> (w1433:T16)
        n895 = case shown="假" w1431 {
          tunnel: w1454 -> [w1496 _]
          tunnel: w1434 -> [w1494 _]
          tunnel: w1433 -> [w1493 w1633]
          frame False {
            # "量程切换前"
            n896 = case shown="\"自动切换测一次\"" "自动切换量程" {
              tunnel: w1496 -> [_ w1509 w1538]
              tunnel: w1494 -> [_ w1505 w1537]
              tunnel: w1493 -> [w1497 w1501 w1536]
              frame "关闭", Default {
                # "关闭自动切换量程"
                n897 = local write "枚举"(enum16{"读取数据", "写入数据", "读取写入DATABASE", "读取参数"}."读取数据" ("枚举")) -> ()
                n898 = call "存数据cloumns(子VI).vi"() -> ("数组"=w1499:string[])  [unwired: 11 in]
                n899 = global write "COD读取DATA全局.vi" "data"(w1497) -> ()
                n900 = call "数据写入database.vi"("data"=w1497, "columns"=w1499, "table"="CODMn") -> ()  [unwired: 8 in, 1 out]
              }
              frame "自动切换测一次" {
                # "自动切换量程选择是否重测"
                n901 = global read "COD测量模式全局.vi" "测量模式"() -> (w1508:string)
                n902 = Not Equal?(x=w1508, y="水样测试") -> (x != y?=w1506:bool)
                n903 = case shown="假" w1506 {
                  tunnel: [w1511 w1512] -> w1504
                  tunnel: w1505 -> [w1511 _]
                  frame False {
                  }
                  frame True {
                    n904 = global read "COD读取DATA全局.vi" "测量数据区"() -> (w1513:T2)
                    n905 = Unbundle By Name(w1513) -> ("水样实测值"=w1512:sgl)
                  }
                }
                n906 = local read "基本量程"() -> (w1510:enum16{"10mg/L", "20mg/L"})
                n907 = case shown="\"20mg/L\"" w1510 {
                  tunnel: w1509 -> [w1515 w1526]
                  tunnel: w1504 -> [w1514 w1525]
                  frame "10mg/L", Default {
                    n908 = Greater?(x=w1514, y="低切高阈值") -> (0:w1516:bool)
                    n909 = case shown="真" w1516 {
                      tunnel: w1515 -> [_ w1519]
                      frame False {
                        n910 = local write "枚举"(enum16{"读取数据", "写入数据", "读取写入DATABASE", "读取参数"}."读取数据" ("枚举")) -> ()
                      }
                      frame True {
                        n911 = local write "枚举"(enum16{"读取数据", "写入数据", "读取写入DATABASE", "读取参数"}."写入数据" ("枚举")) -> ()
                        n912 = Bundle By Name(cluster=cluster{"starting address":u16, "values":u16[]} {"starting address"=0, "values"=[]}, "starting address"=u16 4276, "values"=u16[] [1]) -> (w1521:cluster{"starting address":u16, "values":u16[]})
                        n913 = Enqueue Element(queue=w1519, element=w1521) -> ()  [unwired: 2 in, 3 out]
                      }
                    }
                  }
                  frame "20mg/L" {
                    n914 = Less?(x=w1525, y="高切低阈值") -> (x < y?=w1527:bool)
                    n915 = case shown="真" w1527 {
                      tunnel: w1526 -> [_ w1530]
                      frame False {
                        n916 = local write "枚举"(enum16{"读取数据", "写入数据", "读取写入DATABASE", "读取参数"}."读取数据" ("枚举")) -> ()
                      }
                      frame True {
                        n917 = local write "枚举"(enum16{"读取数据", "写入数据", "读取写入DATABASE", "读取参数"}."写入数据" ("枚举")) -> ()
                        n918 = Bundle By Name(cluster=cluster{"starting address":u16, "values":u16[]} {"starting address"=0, "values"=[]}, "starting address"=u16 4276, "values"=u16[] [0]) -> (w1532:cluster{"starting address":u16, "values":u16[]})
                        n919 = Enqueue Element(queue=w1530, element=w1532) -> ()  [unwired: 2 in, 3 out]
                      }
                    }
                  }
                }
                n920 = call "存数据cloumns(子VI).vi"() -> ("数组"=w1503:string[])  [unwired: 11 in]
                n921 = global write "COD读取DATA全局.vi" "data"(w1501) -> ()
                n922 = call "数据写入database.vi"("data"=w1501, "columns"=w1503, "table"="CODMn") -> ()  [unwired: 8 in, 1 out]
              }
              frame "自动切换测两次" {
                # "自动切换量程选择是否重测"
                n923 = local read "基本量程"() -> (w1539:enum16{"10mg/L", "20mg/L"})
                n924 = case shown="\"10mg/L\", 默认" w1539 {
                  tunnel: w1538 -> [w1543 w1589]
                  tunnel: w1537 -> [w1541 w1587]
                  tunnel: w1536 -> [w1540 w1586]
                  frame "10mg/L", Default {
                    n925 = local read "低切高阈值"() -> (w1542:dbl)
                    n926 = Greater?(x=w1541, y=w1542) -> (0:w1544:bool)
                    n927 = case shown="真" w1544 {
                      tunnel: w1543 -> [_ w1560]
                      tunnel: w1540 -> [w1545 _]
                      frame False {
                        n928 = local write "枚举"(enum16{"读取数据", "写入数据", "读取写入DATABASE", "读取参数"}."读取数据" ("枚举")) -> ()
                        n929 = call "存数据cloumns(子VI).vi"() -> ("数组"=w1547:string[])  [unwired: 11 in]
                        n930 = global write "COD读取DATA全局.vi" "data"(w1545) -> ()
                        n931 = call "数据写入database.vi"("data"=w1545, "columns"=w1547, "table"="CODMn") -> ()  [unwired: 8 in, 1 out]
                      }
                      frame True {
                        n932 = local read "量程切换次数"() -> (w1549:u8)
                        n933 = local write "枚举"(enum16{"读取数据", "写入数据", "读取写入DATABASE", "读取参数"}."写入数据" ("枚举")) -> ()
                        n934 = Increment(x=w1549) -> (x+1=w1550:u8)
                        n935 = local write "量程切换次数"(w1550) -> ()
                        n936 = Bundle By Name(cluster=cluster{"starting address":u16, "values":u16[]} {"starting address"=0, "values"=[]}, "starting address"=u16 4276, "values"=u16[] [1]) -> (w1562:cluster{"starting address":u16, "values":u16[]})
                        n937 = local read "测量模式数字"() -> (w1556:i32)
                        n938 = Enqueue Element(queue=w1560, element=w1562) -> (queue out=w1559:refnum<queue>)  [unwired: 2 in, 2 out]
                        n939 = case shown="0" w1556 {
                          tunnel: [u16 4608 ("address") u16 4608 ("address") u16 4608 ("address") u16 4608 ("address") u16 4608 ("address") u16 4608 ("address") u16 4608 ("address") u16 4608 ("address") u16 4608 ("address") u16 4608 ("address")] -> w1555
                          tunnel: [u16 1 ("address") u16 2 ("address") u16 3 ("address") u16 4 ("address") u16 5 ("address") u16 7 ("address") u16 6 ("address") u16 8 ("address") u16 9 ("address") u16 0 ("address")] -> w1552
                          frame 0 {
                          }
                          frame 1 {
                          }
                          frame 2 {
                          }
                          frame 3 {
                          }
                          frame 4 {
                          }
                          frame 5 {
                          }
                          frame 6 {
                          }
                          frame 7 {
                          }
                          frame 8 {
                          }
                          frame 9, Default {
                          }
                        }
                        n940 = Insert Into Array(array=u16[] [] ("values"), index=0 ("索引"), new element=w1552) -> (w1551:u16[])
                        n941 = Bundle By Name(cluster=cluster{"starting address":u16, "values":u16[]} {"starting address"=0, "values"=[]}, "starting address"=w1555, "values"=w1551) -> (w1558:cluster{"starting address":u16, "values":u16[]})
                        n942 = Enqueue Element(queue=w1559, element=w1558) -> ()  [unwired: 2 in, 3 out]
                      }
                    }
                  }
                  frame "20mg/L" {
                    n943 = local read "高切低阈值"() -> (w1588:dbl)
                    n944 = Less?(x=w1587, y=w1588) -> (x < y?=w1590:bool)
                    n945 = case shown="真" w1590 {
                      tunnel: w1589 -> [_ w1606]
                      tunnel: w1586 -> [w1591 _]
                      frame False {
                        n946 = local write "枚举"(enum16{"读取数据", "写入数据", "读取写入DATABASE", "读取参数"}."读取数据" ("枚举")) -> ()
                        n947 = call "存数据cloumns(子VI).vi"() -> ("数组"=w1593:string[])  [unwired: 11 in]
                        n948 = global write "COD读取DATA全局.vi" "data"(w1591) -> ()
                        n949 = call "数据写入database.vi"("data"=w1591, "columns"=w1593, "table"="CODMn") -> ()  [unwired: 8 in, 1 out]
                      }
                      frame True {
                        n950 = local read "量程切换次数"() -> (w1595:u8)
                        n951 = local write "枚举"(enum16{"读取数据", "写入数据", "读取写入DATABASE", "读取参数"}."写入数据" ("枚举")) -> ()
                        n952 = Increment(x=w1595) -> (x+1=w1596:u8)
                        n953 = Bundle By Name(cluster=cluster{"starting address":u16, "values":u16[]} {"starting address"=0, "values"=[]}, "starting address"=u16 4276, "values"=u16[] [0]) -> (w1608:cluster{"starting address":u16, "values":u16[]})
                        n954 = local write "量程切换次数"(w1596) -> ()
                        n955 = local read "测量模式数字"() -> (w1602:i32)
                        n956 = Enqueue Element(queue=w1606, element=w1608) -> (queue out=w1605:refnum<queue>)  [unwired: 2 in, 2 out]
                        n957 = case shown="0" w1602 {
                          tunnel: [u16 4608 ("address") u16 4608 ("address") u16 4608 ("address") u16 4608 ("address") u16 4608 ("address") u16 4608 ("address") u16 4608 ("address") u16 4608 ("address") u16 4608 ("address") u16 4608 ("address")] -> w1599
                          tunnel: [u16 1 ("address") u16 2 ("address") u16 3 ("address") u16 4 ("address") u16 5 ("address") u16 7 ("address") u16 6 ("address") u16 8 ("address") u16 9 ("address") u16 0 ("address")] -> w1598
                          frame 0 {
                          }
                          frame 1 {
                          }
                          frame 2 {
                          }
                          frame 3 {
                          }
                          frame 4 {
                          }
                          frame 5 {
                          }
                          frame 6 {
                          }
                          frame 7 {
                          }
                          frame 8 {
                          }
                          frame 9, Default {
                          }
                        }
                        n958 = Insert Into Array(array=u16[] [] ("values"), index=0 ("索引"), new element=w1598) -> (w1597:u16[])
                        n959 = Bundle By Name(cluster=cluster{"starting address":u16, "values":u16[]} {"starting address"=0, "values"=[]}, "starting address"=w1599, "values"=w1597) -> (w1604:cluster{"starting address":u16, "values":u16[]})
                        n960 = Enqueue Element(queue=w1605, element=w1604) -> ()  [unwired: 2 in, 3 out]
                      }
                    }
                  }
                }
              }
            }
          }
          frame True {
            # "防止无限切量程"
            n961 = local write "枚举"(enum16{"读取数据", "写入数据", "读取写入DATABASE", "读取参数"}."读取数据" ("枚举")) -> ()
            n962 = local write "量程切换次数"(u8 0 ("量程切换次数")) -> ()
            n963 = call "存数据cloumns(子VI).vi"() -> ("数组"=w1635:string[])  [unwired: 11 in]
            n964 = global write "COD读取DATA全局.vi" "data"(w1633) -> ()
            n965 = call "数据写入database.vi"("data"=w1633, "columns"=w1635, "table"="CODMn") -> ()  [unwired: 8 in, 1 out]
          }
        }
        n966 = global read "COD测量模式全局.vi" "测量模式"() -> (w1446:string)
        n967 = global write "COD浓度全局变量.vi" "COD浓度（mg/L)"(w1434) -> ()
        n968 = Equal?(x=w1446, y="校标") -> (x = y?=w1444:bool)
        n969 = case shown="真" w1444 {
          tunnel: w1453 -> [_ w1675]
          frame False {
          }
          frame True {
            n970 = local read "当前校准"() -> (w1676:i32)
            n971 = case shown="3" w1676 {
              tunnel: w1675 -> [w1677 w1678 w1679 w1680 w1681]
              frame 1, Default {
                n972 = local write "泵滴定数1"(w1677) -> ()
              }
              frame 2 {
                n973 = local write "泵滴定数2"(w1678) -> ()
              }
              frame 3 {
                n974 = local write "泵滴定数3"(w1679) -> ()
              }
              frame 4 {
                n975 = local write "泵滴定数4"(w1680) -> ()
              }
              frame 5 {
                n976 = local write "泵滴定数5"(w1681) -> ()
              }
            }
          }
        }
      }
      frame "读取参数" {
        n977 = Dequeue Element(queue=w1697, timeout in ms (-1)=1000 ("超时毫秒(-1)"), error in (no error)=w1696) -> (element=w1703:T5)  [unwired: 3 out]
        n978 = local write "枚举"(enum16{"读取数据", "写入数据", "读取写入DATABASE", "读取参数"}."读取数据" ("枚举")) -> ()
        n979 = Unbundle By Name(w1703) -> ("starting address"=w1702:u16, "number of holding registers"=w1701:u16)
        n980 = local read "读取KB值"() -> (w1692:bool)
        n981 = call <vilib>:"Read Holding Registers.vi"("error in (no error)"=w1698, "quantity"=w1701, "starting address"=w1702, "MB session in"=w1699) -> ("error out"=w1691:errorcluster, "Registers"=w1695:u16[], "MB session out"=w1693:refnum<class "MB_Master_Serial.lvclass">)  [unwired: 5 in]
        n982 = case shown="假" w1692 {
          tunnel: w1695 -> [w1715 w1738]
          tunnel: w1691 -> [_ w1740]
          frame False {
            n983 = Index Array(array=w1715) -> (element #1=w1709:u16, element #2=w1726:u16, element #3=w1725:u16, element #4=w1707:u16, element #5=w1705:u16, element #6=w1704:u16, element #7=w1724:u16, element #8=w1723:u16, element #9=w1722:u16, element #10=w1721:u16, element #11=w1720:u16, element #12=w1719:u16, element #13=w1718:u16, element #14=w1717:u16, element #15=w1716:u16, element #16=w1714:u16)  [unwired: 16 in]
            n984 = local write "硫酸"(w1718) -> ()
            n985 = local write "标液"(w1723) -> ()
            n986 = Divide(x=w1709, y=u16 10) -> (x/y=w1710:dbl)
            n987 = local write "草酸钠"(w1719) -> ()
            n988 = local write "蒸馏水"(w1724) -> ()
            n989 = local write "质控样"(w1722) -> ()
            n990 = local write "加标回收"(w1721) -> ()
            n991 = local write "高锰酸钾"(w1720) -> ()
            n992 = local write "零点泵计量数 2"(w1717) -> ()
            n993 = local write "标度泵计量数 2"(w1716) -> ()
            n994 = local write "水样"(w1704) -> ()
            n995 = Divide(x=w1707, y=u16 100) -> (x/y=w1706:dbl)
            n996 = Divide(x=w1714, y=u16 100) -> (x/y=w1713:dbl)
            n997 = local write "恒温时间"(w1726) -> ()
            n998 = local write "浓度"(w1725) -> ()
            n999 = local write "温度"(w1710) -> ()
            n1000 = local write "基本量程"(w1705) -> ()
            n1001 = local write "修正系数 2"(w1706) -> ()
            n1002 = local write "浓度 2"(w1713) -> ()
          }
          frame True {
            (unwired) 9 ("索引")
            n1003 = case shown="错误" w1740 {
              tunnel: ["读取成功" ("消息") "读取失败" ("消息")] -> w1739
              frame No Error {
              }
              frame Error {
              }
            }
            n1004 = Array Subset(array=w1738, index=10 ("索引"), length=18 ("长度")) -> (w1735:u16[])
            n1005 = call "浮点CDAB转换COD.vi"("数组"=w1735) -> ("数组 2"=w1734:sgl[])  [unwired: 10 in]
            n1006 = One Button Dialog(message=w1739) -> ()  [unwired: 1 in, 1 out]
            n1007 = Array To Cluster(array=w1734) -> (cluster=w1733:T18)
            n1008 = local read "量程选择"() -> (w1727:enum16{"低量程", "高量程", "0-2量程"})
            n1009 = case shown="\"0-2量程\"" w1727 {
              tunnel: w1733 -> [w1744 w1748 w1752]
              tunnel: [w1743 w1747 w1751] -> w1730
              tunnel: [w1742 w1746 w1750] -> w1729
              tunnel: [w1741 w1745 w1749] -> w1728
              frame "低量程", Default {
                n1010 = Unbundle By Name(w1744) -> ("数组 2[2]"=w1743:sgl, "数组 2[0]"=w1742:sgl, "数组 2[1]"=w1741:sgl)
              }
              frame "高量程" {
                n1011 = Unbundle By Name(w1748) -> ("数组 2[5]"=w1747:sgl, "数组 2[3]"=w1746:sgl, "数组 2[4]"=w1745:sgl)
              }
              frame "0-2量程" {
                n1012 = Unbundle By Name(w1752) -> ("数组 2[8]"=w1751:sgl, "数组 2[6]"=w1750:sgl, "数组 2[7]"=w1749:sgl)
              }
            }
            n1013 = Bundle By Name(cluster=cluster{"X^2":dbl, "X":dbl, "b":dbl} {"X^2"=0.0, "X"=0.0, "b"=0.0} ("方程系数"), "X^2"=w1730, "X"=w1729, "b"=w1728) -> (w1731:cluster{"X^2":dbl, "X":dbl, "b":dbl})
            n1014 = local write "方程系数"(w1731) -> ()
          }
        }
      }
    }
    n1015 = Unbundle By Name(w1342) -> ("status"=w1343:bool)
    n1016 = Not(x=w1343) -> (.not. x?=→"通讯状态":bool)
  }
  n1017 = call-dynamic "Close Session.vi"("error in (no error)"=w30, "MB_Serial session"=w29) -> ()  [unwired: 9 in, 1 out]
  "COM" <- "VISA resource name"
